vi "LBCB Operation Manager.vi"() -> ()   [LabVIEW 2009]
uses:
  lib/Data Display/External Sensor Name & Value.ctl
  lib/Data Access Objects/Application/App Parameters.ctl
  lib/Data Access Objects/Application/Timing Parameters.ctl
  lib/Apps/AppStates.ctl
  lib/Data Access Objects/Metadata/LBCB Number.ctl
  lib/Data Access Objects/Metadata/LBCB Location.ctl
  lib/Data Access Objects/Control Loop/PID Controls.ctl
  lib/Apps/Lbcb Control Loop States.ctl
  lib/MixedMode/Stiffness Matrix.ctl
  lib/MixedMode/Target Data.ctl
  lib/MixedMode/Mixed Mode Cartesian Data.ctl
  lib/MixedMode/Mixed Mode Convergence Status.ctl
  lib/Autobalance/Autobalance Display Data Point.ctl
  lib/Autobalance/Autobalance Stage.ctl
  lib/Apps/Yes No Button.ctl
  lib/Data Access Objects/Autobalance/Autobalance Control Parameters.ctl
  lib/Data Access Objects/Metadata/Actuator Point.ctl
  lib/Data Access Objects/Metadata/Cartesian Force Vector.ctl
  lib/Data Access Objects/Metadata/Cartesian Force Matrix.ctl
  lib/Data Access Objects/Mixed Mode/Force Control Parameters.ctl
  lib/Data Access Objects/Metadata/Cartesian Point.ctl
  lib/MixedMode/Mixed Mode States.ctl
  lib/MixedMode/Mixed Mode Multidof State.ctl
  lib/Apps/App Parameters Actions.ctl
  lib/Apps/App Status Actions.ctl
  lib/Apps/GUI Control.ctl
  lib/MixedMode/Messages/MM Widget Parameter Changes.ctl
  lib/Control Loop/Parameters Changes.ctl
  lib/Control Loop/Parameter Change States.ctl
  lib/MixedMode/Messages/Mixed Mode Command.ctl
  lib/MixedMode/Mixed Mode Command Action.ctl
  lib/MixedMode/Ramp Time Tuple.ctl
  lib/Data Access Objects/Metadata/Persistant DAO Actions.ctl
  lib/MixedMode/Messages/Mixed Mode Status.ctl
  lib/Data Access Objects/Metadata/DAO Actions.ctl
  lib/Data Access Objects/Application/Number Of LBCBs.ctl
  lib/Limits/Faults List Actions.ctl
  lib/Configuration/ConfigPathActions.ctl
  lib/Launcher/Launcher Actions.ctl
  lib/Logging/Log Filename Actions.ctl
  lib/Launcher/NoPanelAppTypes.ctl
  lib/Global Data/Actuator Measurment Actions.ctl
  lib/Logging/LogFileType.ctl
  lib/Global Data/Cartesian Measurment Actions.ctl
  lib/DAQ IO/Daq Actions.ctl
  lib/Control Loop/LBCB_Conversions_Actions.ctl
panel:
  out "Rigid Connection":T1
  in  "Snapshot":bool
  out "LBCB  Location Out":T2
  in  "Start AB Selected":bool
  in  "Start Autobalance":bool
  in  "Fake":bool
  out "LBCB 2 State":T3
  out "LBCB 1 State":T3
  in  "LBCB Number Button":bool
  in  "L2 Control":bool caption="LBCB 2"
  in  "L1 Control":bool caption="LBCB 1"
  out "L2 Force Limit":bool=TRUE caption="Force"
  out "L2 Displacement Limit":bool=TRUE caption="Displacement"
  out "L2 Auto Balance":bool=TRUE caption="Auto Balance"
  in  "PID Control":T4={"I-Control"=TRUE, "Ctrl Mode"=TRUE}
  in  "LBCB Number":T5
  out "State":T6=enum."Initializing Displays"
  out "Application Timing and Logging":T7
  out "External Sensor Names":string[](array[string])
  out "all stopped":bool
  out "Messages":string
  out "L1 Force Limit":bool=TRUE caption="Force"
  out "L1 Displacement Limit":bool=TRUE caption="Displacement"
  out "L1 Auto Balance":bool=TRUE caption="Auto Balance"
  in  "stop":bool
  in  "Monitor Panel":T9(tab)
  out "Cartesian DOF Labels":string[](array[string])=["X", "Y", "Z", "Rx", "Ry", "Rz"]
  out "Cartesian Space Labels":string[](array[string])=["Commands (in/rad)", "Displacements (in/rad)", "Forces (lbs/lb*in)"]
  out "External Sensors":T10[](array[typedef])
  out "Cartesian Digital Display Table":dbl[][](array[numeric])
  out "Actuator Digital Display":dbl[][](array[numeric])
  out "Actuator DOF Labels":string[](array[string])=["X1", "X2", "Y1", "Z1", "Z2", "Z3"]
  out "Actuator Space Labels":string[](array[string])=["Commands (in/rad)", "Displacements (in/rad)", "Forces (lbs/lb*in)"]
  out "Actuator X1":dbl(slide)=0.012801822908652838 step=0.0005 scale=-10.0..10.0
  out "Actuator X2":dbl(slide)=0.012801822908652838 step=0.0005 scale=-10.0..10.0
  out "Actuator Y1":dbl(slide)=7.98290599846041e-06 step=0.0005 scale=-5.0..5.0
  out "Actuator Z1":dbl(slide)=8.154359441903125e-06 step=0.0005 scale=-5.0..5.0
  out "Actuator Z2":dbl(slide)=8.154359441903125e-06 step=0.0005 scale=-5.0..5.0
  out "Actuator Z3":dbl(slide)=8.154359441903125e-06 step=0.0005 scale=-5.0..5.0
  in  "Cartesian Type":bool caption="Coord"
  out "External Sensors Volts":T10[](array[typedef]) caption="External Sensor Voltages"
  out "Actuator Labels":string[](array[string])=["X1", "X2", "Y1", "Z1", "Z2", "Z3"]
  out "Voltage Labels":string[](array[string])=["Commands", "LVDTs", "Load Cells", "Servo Errors"]
  out "Raw Data":dbl[][](array[numeric])
  in  "Force Error Range":T11
  in  "Jacobian Gain":T12
  in  "Max Increment":T12
  in  "Force Control Parameters":T13
  in  "Stiffness Limit":T14
  in  "Force Group Priorities":T11
  out "Convergence":T15
  out "Measurements":T16
  out "Target":T17
  in  "Stiffness Jacobian":T18=[[1000000.0, 0.0, 0.0, 0.0, 0.0, 0.0], [0.0, 1000000.0, 0.0, 0.0, 0.0, 0.0], [0.0, 0.0, 1000000.0, 0.0, 0.0, 0.0], [0.0, 0.0, 0.0, 1000000.0, 0.0, 0.0], [0.0, 0.0, 0.0, 0.0, 1000000.0, 0.0], [0.0, 0.0, 0.0, 0.0, 0.0, 1000000.0]]
  out "MixedModeStates":T19
  out "Mixed Mode Multidof State":T20
  out "MM Multi Ramp Count":i32 caption="Ramp Count"
  out "Stiffness Tested":T1[](array[typedef])
  in  "Auto Balance Error Window":T21
  in  "Auto Balance Control":T22={"Number of Samples"=0, "Delay After Cmd"=0, "Maximum Command"=0.0, "1/4 Linear Range"=0.5}
  out "Autobalance Statuses":T23[](array[typedef])
  out "Logo":picture
  # "Operations Manager"
  # "Ver 3.2.0"
  # "NEES MUST-SIM Facility"
  # "University of Illinois at Urbana-Champaign"
  # "Control"
  # "Continuous"
  # "Hold"
  # "Interval is in Seconds\nRate is in Samples per Second"
  # "(inch)"
  # "(inch)"
  # "(inch)"
  # "(inch)"
  # "(inch)"
  # "(inch)"
  # "Actuator\nSpace"
  # "Name"
  # "Cartesian\nSpace"
  # "Multi DOF\nStatus"
  # "(Volts)"
  # "Cmd"
  # "Servo Error"
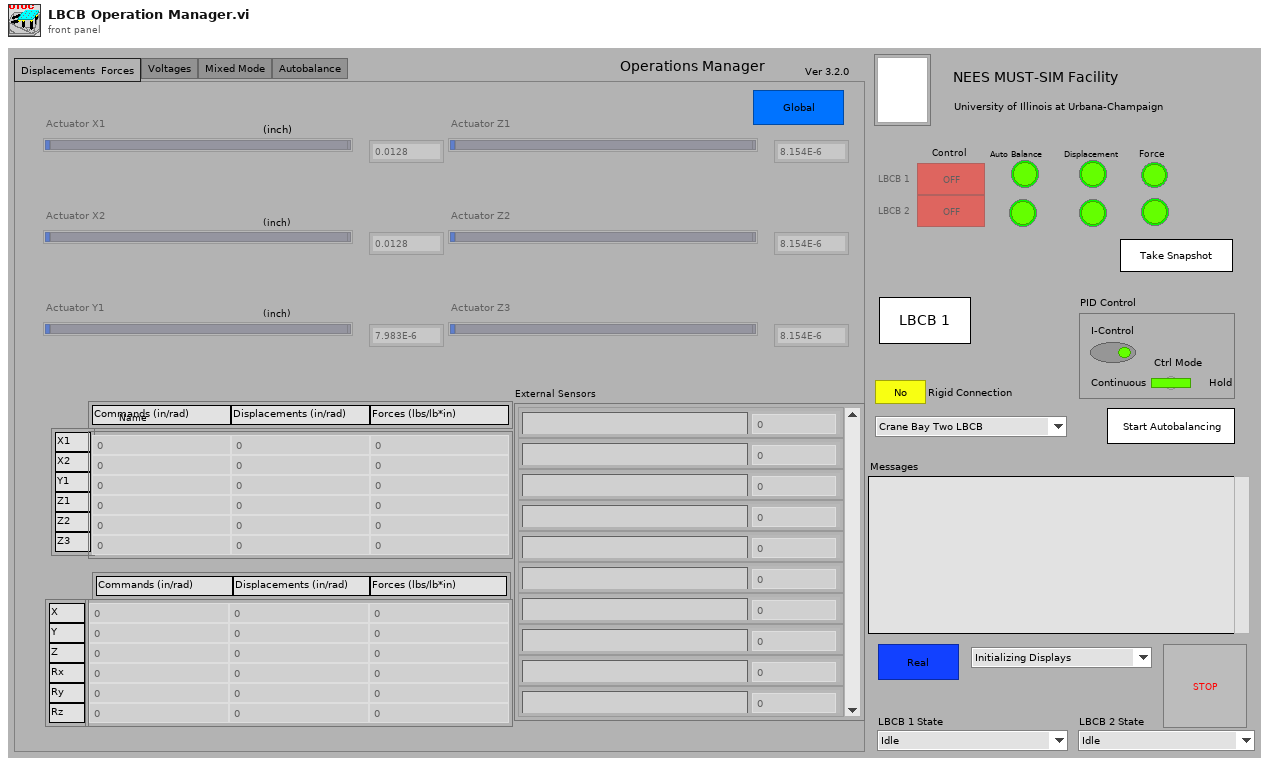
[diagram p1: front panel]
types:
  T1 = typedef "Yes No Button.ctl" = bool
  T2 = typedef "LBCB Location.ctl" = enum16{"Crane Bay Two LBCB", "Crane Bay One LBCB", "5th Scale Two LBCB", "5th Scale One LBCB", "Portable LBCB"}
  T3 = typedef "Lbcb Control Loop States.ctl" = enum16{"Idle", "Start Selected", "Load Last Command", "Start Autobalancing", "Autobalancing", "Control Loop Initialized", "Control Enabled"}
  T4 = typedef "PID Controls.ctl" = cluster{"I-Control":bool, "Ctrl Mode":bool}
  T5 = typedef "LBCB Number.ctl" = enum16{"LBCB1", "LBCB2"}
  T6 = typedef "AppStates.ctl" = enum16{"Starting OM", "Initializing Displays", "Setting up Archiving", "Setting Up DAQ Channels", "Start DAQ", "DAQ Starting", "Controlling LBCBs", "Stopping OM"}
  T7 = typedef "App Parameters.ctl" = cluster{"Monitor Loop":T8, "Ramp Time":T8, "Log Loop":T8, "TCP to DAQ":T8, "Logging Directory":path, "Log File Size (MBytes)":i64, "Volt Logging Loop":T8, "2 LBCB Archiving Mode":bool}
  T8 = typedef "Timing Parameters.ctl" = cluster{"Interval":dbl, "Rate ":dbl}
  T9 = enum32{"Displacements  Forces", "Voltages", "Mixed Mode", "Autobalance"}
  T10 = typedef "External Sensor Name & Value.ctl" = cluster{"Name":string, "Value":dbl}
  T11 = typedef "Cartesian Force Vector.ctl" = cluster{"Fx":dbl, "Fy":dbl, "Fz":dbl, "Mx":dbl, "My":dbl, "Mz":dbl}
  T12 = typedef "Cartesian Point.ctl" = cluster{"Dx":dbl, "Dy":dbl, "Dz":dbl, "Rx":dbl, "Ry":dbl, "Rz":dbl}
  T13 = typedef "Force Control Parameters.ctl" = cluster{"Use Force Error Range Ratios":bool, "Use Group Priorities":bool, "Multi Command Update":bool, "Steps per Stiffness \nMeasurement":i32}
  T14 = typedef "Cartesian Force Matrix.ctl" = cluster{"Lower":T11, "Upper":T11}
  T15 = typedef "Mixed Mode Convergence Status.ctl" = cluster{"IsConverged":bool[], "Force Errors":dbl[], "Controlling DOF":bool[]}
  T16 = typedef "Mixed Mode Cartesian Data.ctl" = cluster{"Displacements":dbl[], "Forces":dbl[]}
  T17 = typedef "Target Data.ctl" = cluster{"Displacements":dbl[], "Command Type":enum16{"<None>", "Displacement", "Force"}[], "Forces":dbl[]}
  T18 = typedef "Stiffness Matrix.ctl" = dbl[][]
  T19 = typedef "Mixed Mode States.ctl" = enum16{"Init", "Wait For DAQ", "Idle", "Start Initial Position", "Initial Position", "Start Initial Ramp", "Run Initial Ramp", "Start Iterative Stage", "Convergence Check", "Update Stiffness Jacobian", "Update Command", "Start Iterative Ramp", "Run Iterative Ramp", "Start Iterative Stabilize", "Iterative Stabilize", "Start Iterative Holding", "Iterative Holding", "Start Stabilize", "Stabilize", "Start Hold", "Holding", "Done", "Aborting", "Exit", "Nop"}
  T20 = typedef "Mixed Mode Multidof State.ctl" = enum16{"Multidof", "Stiffness Test", "Start Iterative Stage"}
  T21 = typedef "Actuator Point.ctl" = cluster{"X1":dbl, "X2":dbl, "Y1":dbl, "Z1":dbl, "Z2":dbl, "Z3":dbl}
  T22 = typedef "Autobalance Control Parameters.ctl" = cluster{"Number of Samples":i32, "Delay After Cmd":i32, "Maximum Command":dbl, "1/4 Linear Range":dbl}
  T23 = typedef "Autobalance Display Data Point.ctl" = cluster{"LoCmd":dbl, "LoServo":dbl, "HiCmd":dbl, "HiServo":dbl, "Autobalance Stage":T24, "IsBalanced":T1}
  T24 = typedef "Autobalance Stage.ctl" = enum16{"Coarse", "Fine", "Backing Up", "Done"}
  T25 = typedef "Mixed Mode Status.ctl" = cluster{"LBCB Target":T17[], "MixedModeStates":T19, "LBCB Convergence":T15[], "LBCB Measurements":T16[]}
  T26 = typedef "GUI Control.ctl" = cluster{"Command":T27, "LBCB Number":enum16{"LBCB1", "LBCB2"}}
  T27 = typedef "MM Widget Parameter Changes.ctl" = enum16{"Start", "Stop All", "Cartesian Type Changed", "Control Enabled", "Control Disabled", "NTCP Link On", "NTCP Link Off"}
  T28 = typedef "Persistant DAO Actions.ctl" = enum16{"Init", "Get", "Set", "Load", "Save"}
  T29 = typedef "Mixed Mode Command.ctl" = cluster{"Command":T30, "Ramp Times":cluster{"Initial":T31, "Iterative":T31}, "LBCB1":T17, "LBCB2":T17}
  T30 = typedef "Mixed Mode Command Action.ctl" = enum16{"Start Command", "Stop", "Exit", "No Op", "Start Acquisition", "Measure Initial Position"}
  T31 = typedef "Ramp Time Tuple.ctl" = cluster{"Ramp":dbl, "Stab":dbl, "Hold":dbl}
  T32 = typedef "Parameters Changes.ctl" = cluster{"Change State":T33, "LBCB Number":T5}
  T33 = typedef "Parameter Change States.ctl" = enum16{"Mixed Mode", "Control Loop", "Limits", "Application", "Stiffness Jacobian", "Start DAQ", "Reset Auto-Balance", "Set Command", "Enable Control", "Disable Control", "Position", "Stop Application"}
  T34 = typedef "App Status Actions.ctl" = enum16{"Init", "Get Status", "Running", "Control", "Autobalanced", "Data Acquisition", "Set App State", "DAQ Started", "Set LBCB State", "Set All", "Set Cont Logging", "Set Step Logging", "Set MM Logging", "Set Volt Logging", "Set Cart Type", "Set DAQ Link", "Set NTCP Link"}
  T35 = enum8{"Enabled", "Disabled", "Disabled and Grayed Out"}
  T36 = typedef "Number Of LBCBs.ctl" = enum16{"1", "2"}
  T37 = typedef "LBCB Settings.ctl" = cluster{"Size":T38, "Type":T39}
  T38 = typedef "LBCB Size.ctl" = enum16{"1/5th-scale LBCB", "Full-scale LBCB", "Portable LBCB"}
  T39 = typedef "LBCB Type.ctl" = enum16{"X Actuators On The Left", "X Actuators On The Right"}
  T40 = typedef "App Parameters Actions.ctl" = enum16{"Init", "Get", "Set"}
  T41 = typedef "DAO Actions.ctl" = enum16{"Init", "Get", "Set"}
  T42 = typedef "NoPanelAppTypes.ctl" = enum16{"NTCP Socket", "Data Archiving", "DAQ Link", "Control Loops", "Cmd Disp Diffs", "Individual Readings", "Limits", "Increment Limits"}
  T43 = typedef "Launcher Actions.ctl" = enum16{"Launch", "Stop All", "Stop", "Kill", "Running?", "Init"}
  T44 = typedef "Cartesian Matrix.ctl" = cluster{"Lower":T12, "Upper":T12}
  T45 = typedef "Faults List Actions.ctl" = enum16{"Init", "Add", "Remove", "Get List"}
  T46 = typedef "ConfigPathActions.ctl" = enum16{"Init", "Application", "MixedMode", "ControlLoop", "Calibration", "System", "Change Location"}
  T47 = typedef "Log Filename Actions.ctl" = enum16{"Init", "Get Filename", "New Log Directory"}
  T48 = typedef "Actuator Measurment Actions.ctl" = enum16{"Set  Data", "Get", "Init"}
  T49 = typedef "LogFileType.ctl" = enum16{"Continuous", "Step", "Volts", "Offsets", "Mixed Mode State", "DLL  Errors", "Snapshot", "End List"}
  T50 = typedef "Daq Actions.ctl" = enum16{"Init", "Send Commands", "Get Responses", "Stop"}
  T51 = typedef "LBCB_Conversions_Actions.ctl" = enum16{"A2C", "C2A", "Set Log Filename", "Init"}
  T52 = typedef "App Status.ctl" = cluster{"Running":bool, "Controlling L2":bool, "Autobalance L2":bool, "Data Acquisition":bool, " App State":T6, "DAQ Started":bool, "LBCB 1 State":T3, "LBCB 2 State":T3, "Controlling L1":bool, "Autobalance L1":bool, "Cartesian Type":bool, "Continuous Logging":bool, "Step Logging":bool, "Voltage Logging":bool, "Mixed Mode Logging":bool, "DAQ Link":bool, "NTCP Link ":bool}
  T53 = typedef "Limit Boundary Parameters.ctl" = cluster{"Lower":dbl, "Upper":dbl, "Label":string}
  T54 = typedef "imagedata.ctl" = cluster{"image type":i32, "image depth":i32, "image":u8[], "mask":u8[], "colors":u32[], "Rectangle":cluster{"left":i16, "top":i16, "right":i16, "bottom":i16}}
  T55 = typedef "Cartesian Measurment Actions.ctl" = enum16{"Set Data", "Get", "Init", "Set Offsets"}
  T56 = typedef "Actuator DataType.ctl" = cluster{"LVDTs":dbl[], " Commands":dbl[], "Load Cells":dbl[], "Servo":dbl[]}
  T57 = typedef "Mixed Mode Multidof Status.ctl" = cluster{"Mixed Mode Multidof State":T20, "Multi DOF Ramp Count":i32, "Stiffness Tested":T1[][]}
  T58 = typedef "Autobalance Status Data.ctl" = cluster{"IsBalanced":T1, "Autobalance Stage":T24, "High":T59, "Low":T59, "Balanced \nCmd":dbl}
  T59 = typedef "Autobalance Data Point.ctl" = cluster{"cCmd":dbl, "cServo":dbl, "pCmd":dbl, "pServo":dbl}
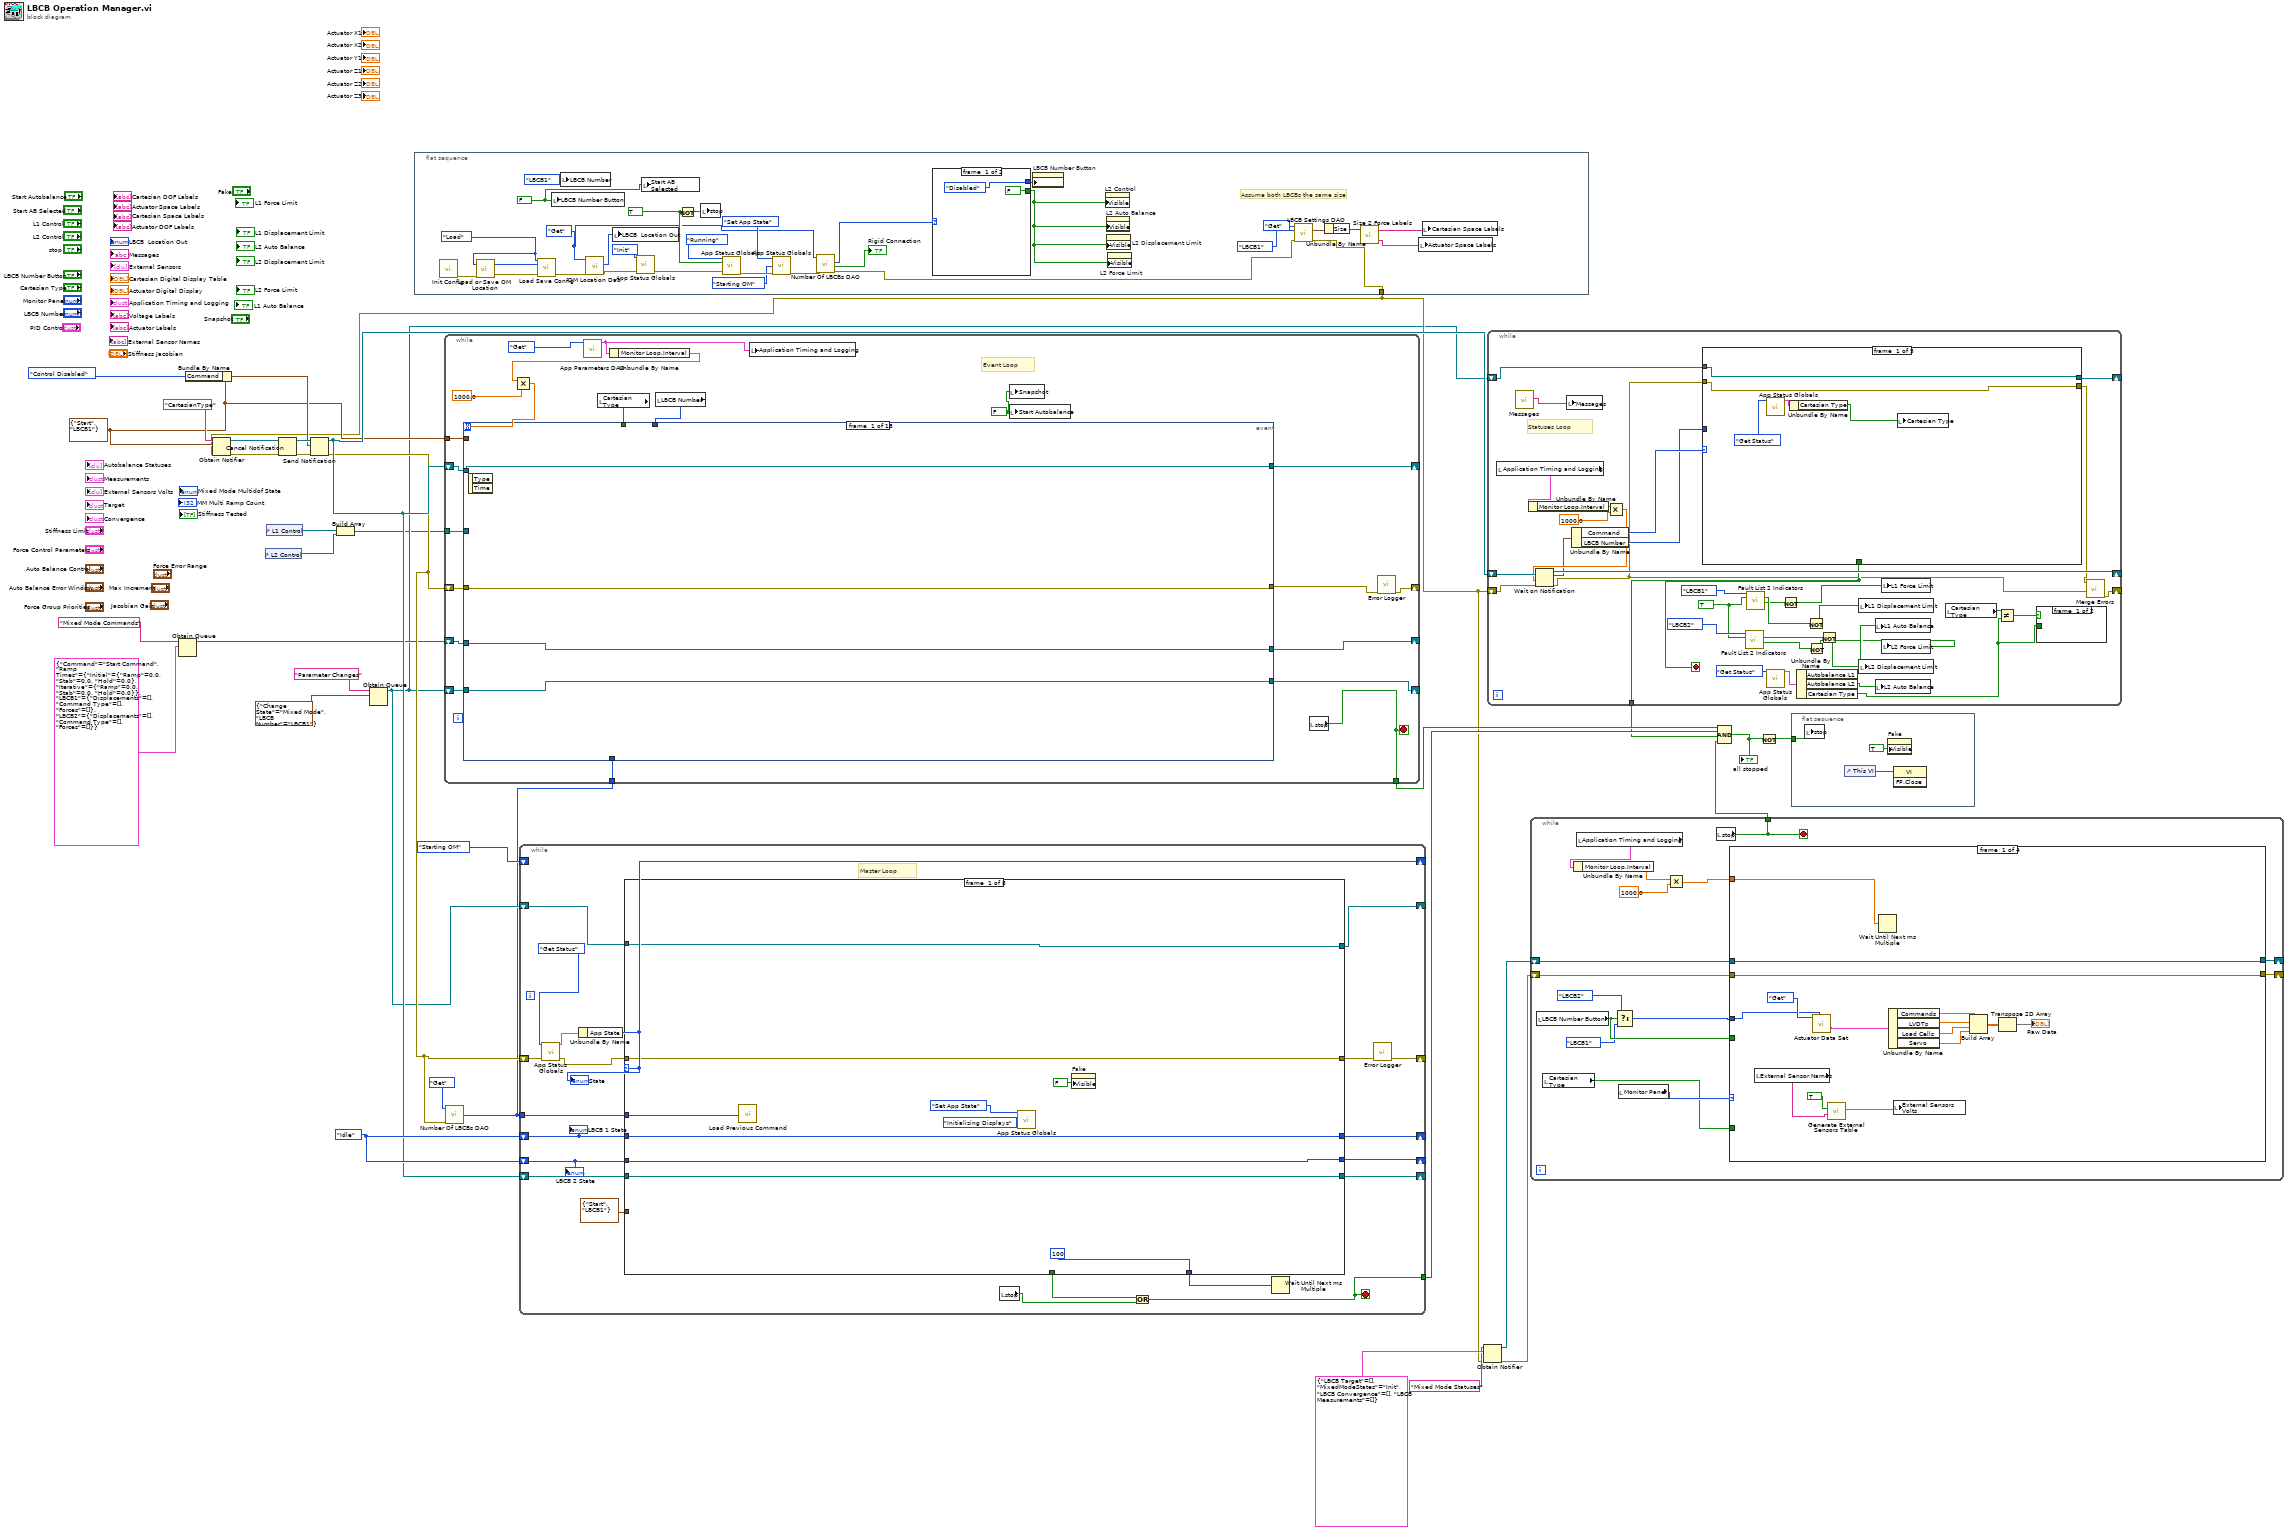
[diagram p0: block diagram]
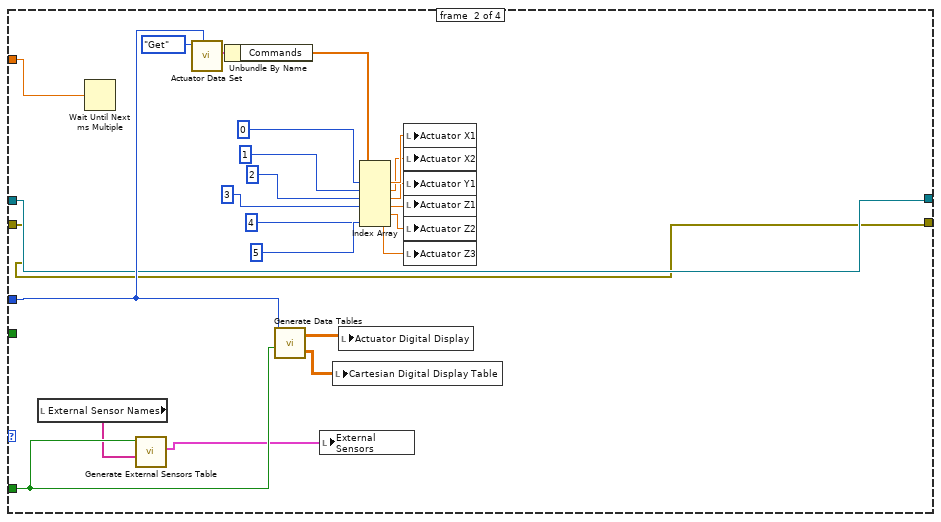
[diagram p2: hidden frame]
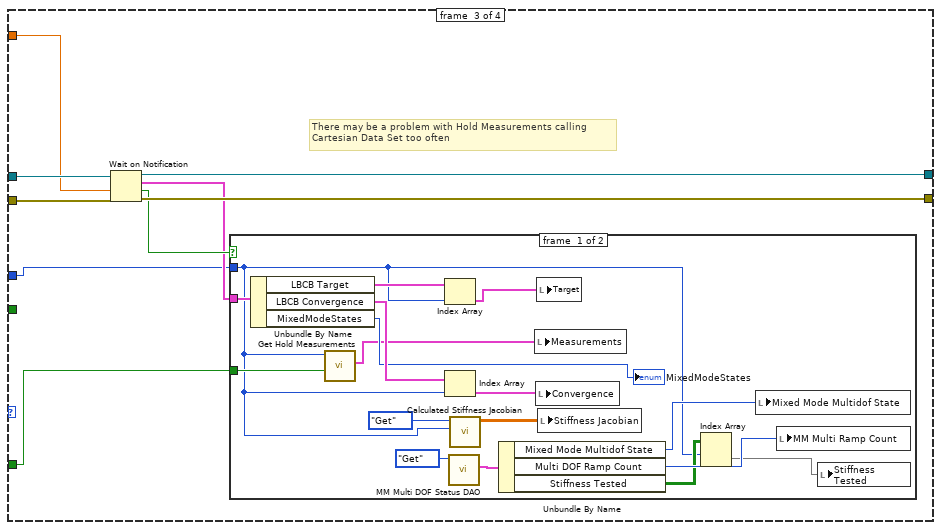
[diagram p3: hidden frame]
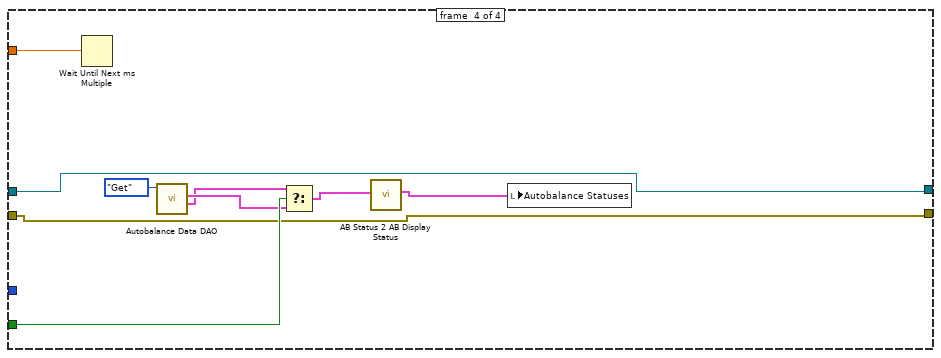
[diagram p5: hidden frame]
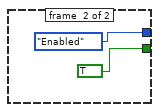
[diagram p6: hidden frame]
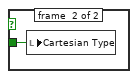
[diagram p7: hidden frame]
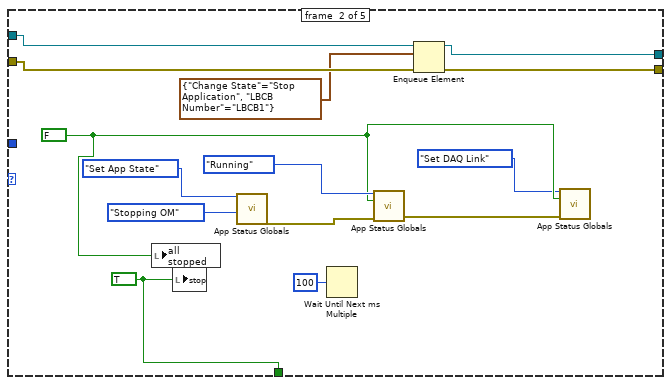
[diagram p8: hidden frame]
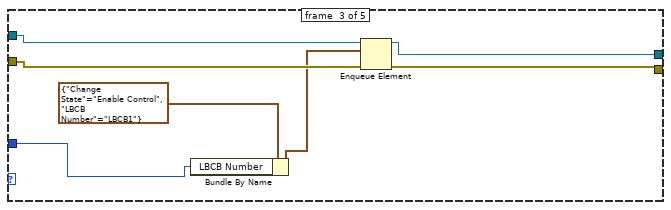
[diagram p9: hidden frame]
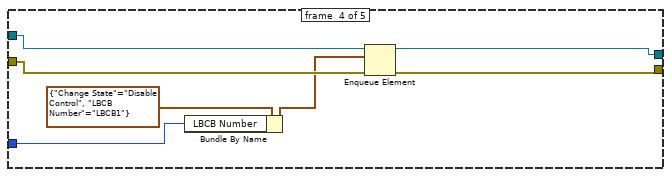
[diagram p10: hidden frame]
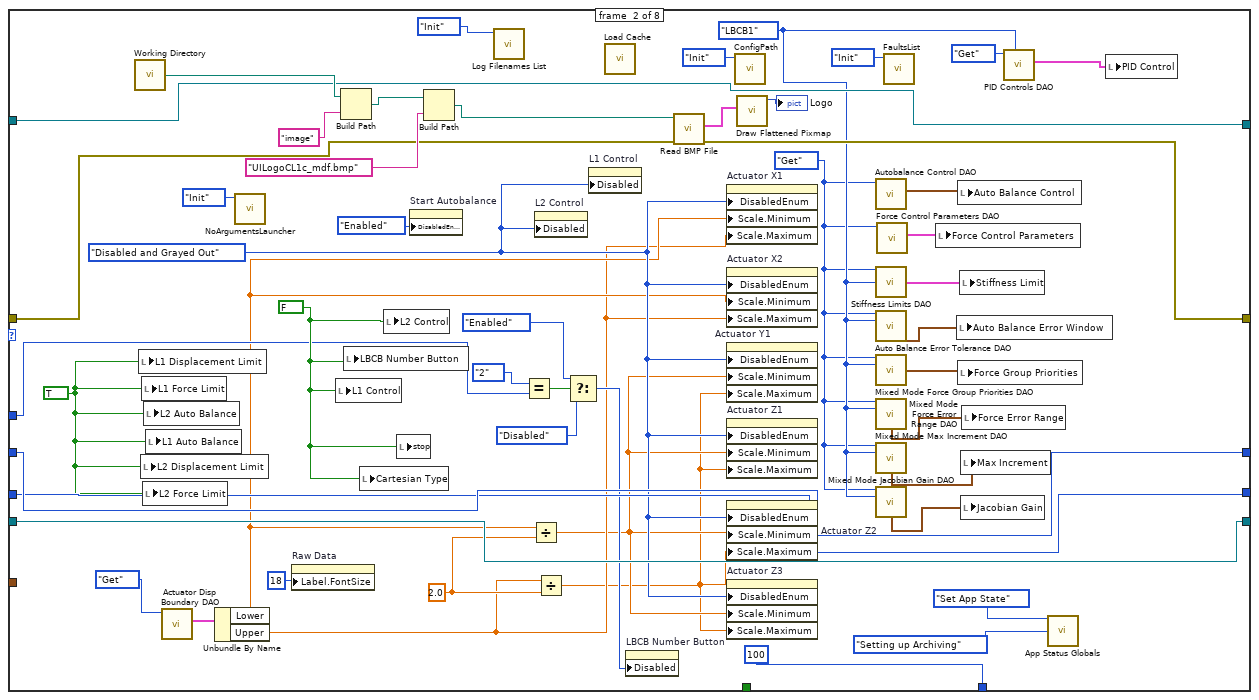
[diagram p12: hidden frame]
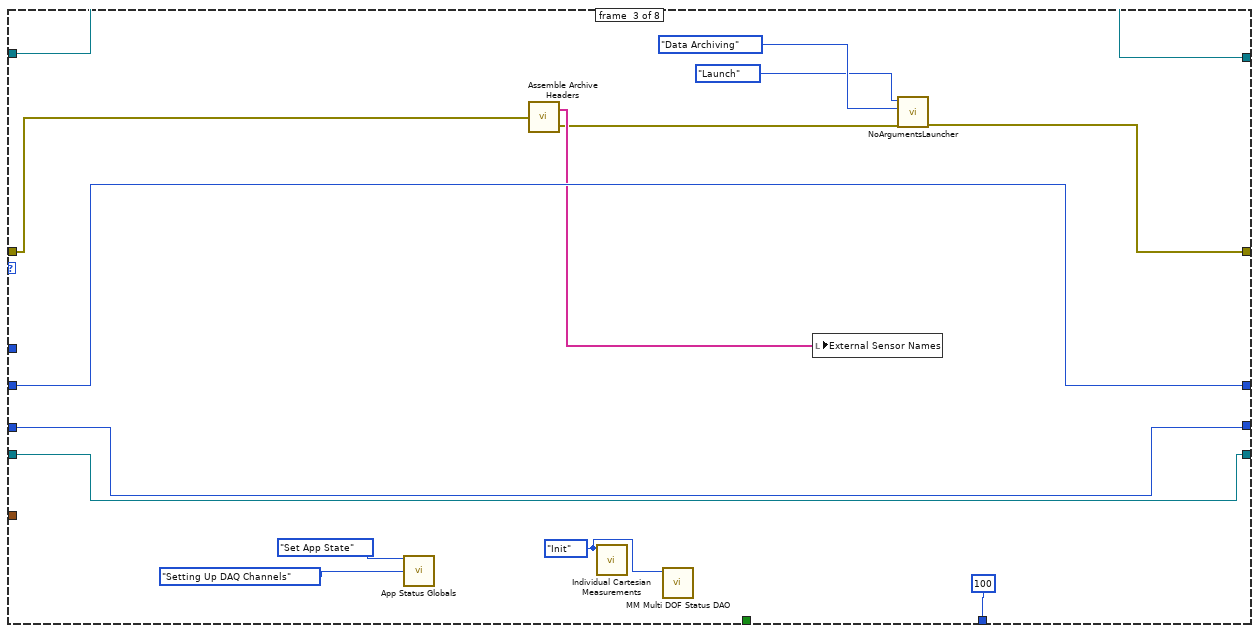
[diagram p13: hidden frame]
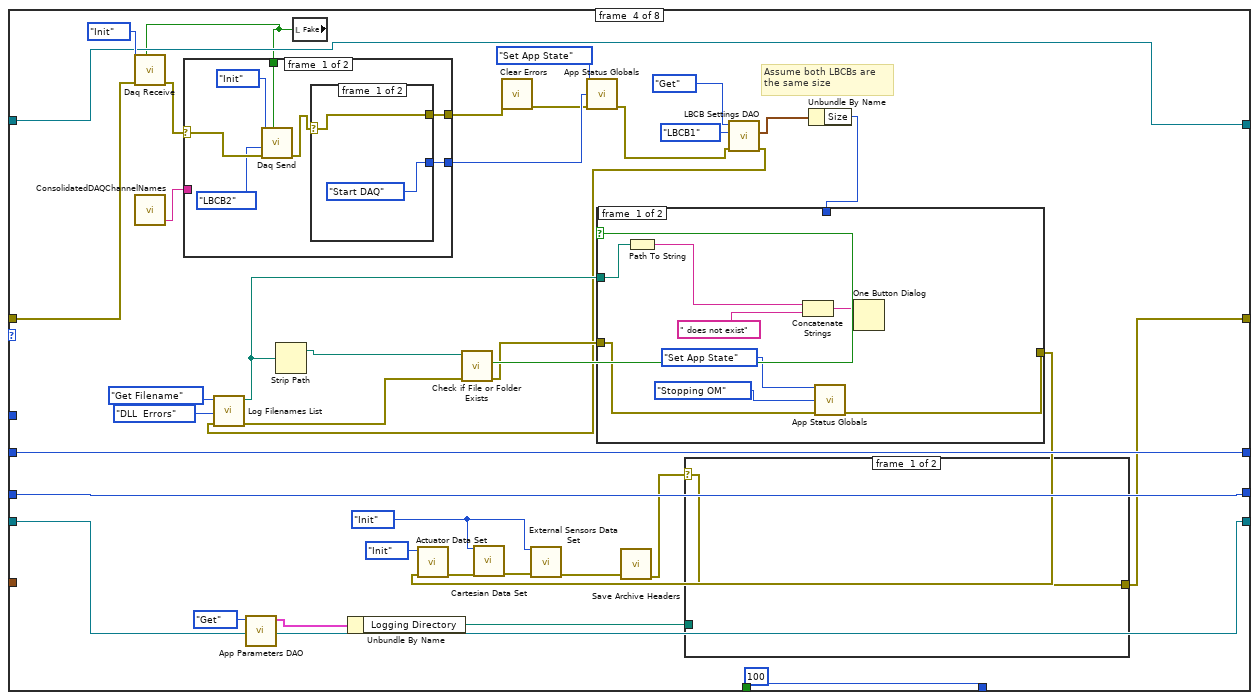
[diagram p14: hidden frame]
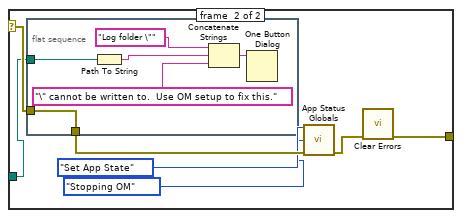
[diagram p15: hidden frame]
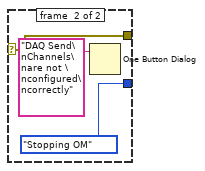
[diagram p16: hidden frame]
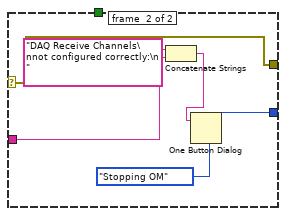
[diagram p17: hidden frame]
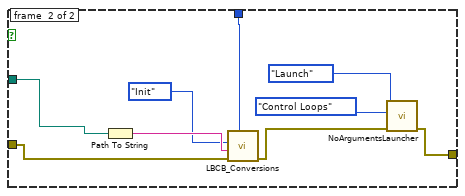
[diagram p18: hidden frame]
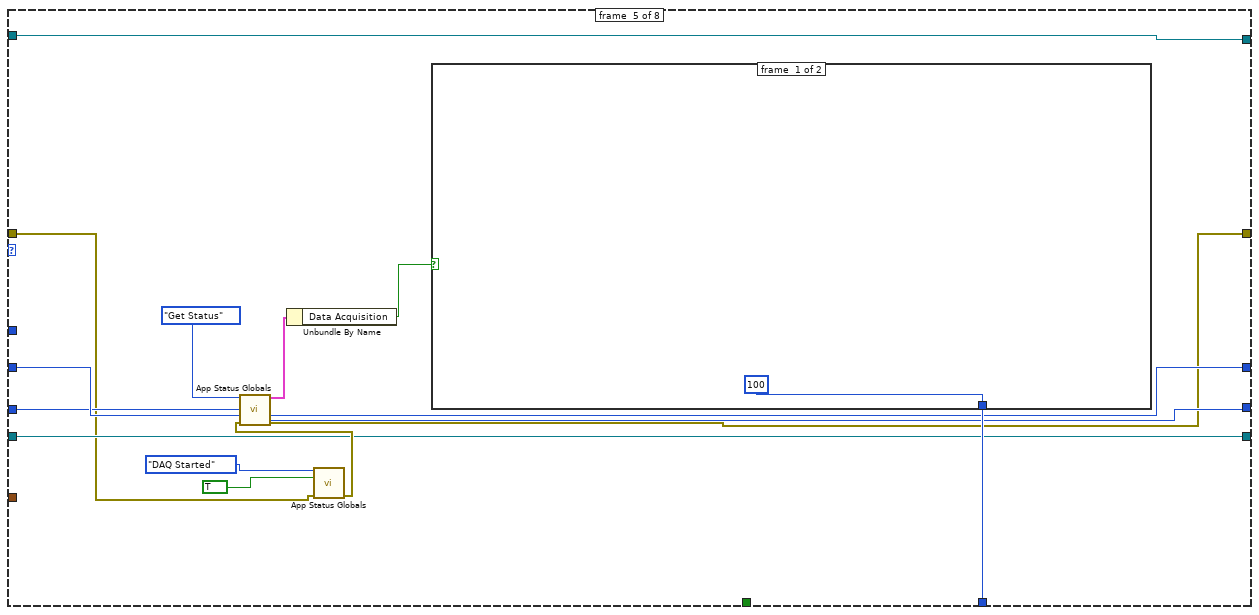
[diagram p19: hidden frame]
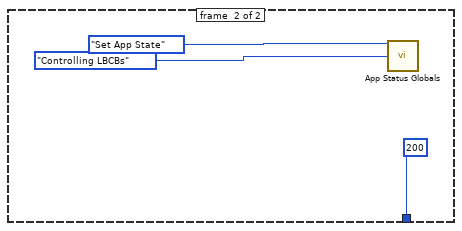
[diagram p20: hidden frame]
diagram:
  w13 = T26 {"Command"=enum."Start", "LBCB Number"=enum."LBCB1"} ("GUI Control")
  w26 = Lbcb_Control_Loop_States."Idle" ("f")
  n1 = Obtain Queue(name (unnamed)="Mixed Mode Commands", element data type=T29 {"Command"=enum."Start Command", "Ramp Times"={"Initial"={"Ramp"=0.0, "Stab"=0.0, "Hold"=0.0}, "Iterative"={"Ramp"=0.0, "Stab"=0.0, "Hold"=0.0}}, "LBCB1"={"Displacements"=[], "Command Type"=[], "Forces"=[]}, "LBCB2"={"Displacements"=[], "Command Type"=[], "Forces"=[]}} ("Mixed Mode Command")) -> (queue out=w6:refnum<queue>)  [unwired: 3 in, 2 out]
  n2 = Bundle By Name(cluster=w13, "Command"=MM_Widget_Parameter_Changes."Control Disabled" ("notification")) -> (w15:T26)
  n3 = Obtain Notifier(name (unnamed)="CartesianType", notification data type=w13, error in (no error)=w7) -> (notifier out=w34:refnum<notifier>, error out=w18:errorcluster)  [unwired: 1 in, 1 out]
  n4 = control-ref of="L2 Control"() -> (w3:refnum<vi>)
  n5 = control-ref of="L1 Control"() -> (w4:refnum<vi>)
  n6 = Cancel Notification(0:w34, 3:w18) -> (8:w20:refnum<notifier>, 11:w17:errorcluster)  [unwired: 1 out]
  n7 = Send Notification(notification=w15, notifier=w20, error in (no error)=w17) -> (notifier out=w19:refnum<notifier>, error out=w16:errorcluster)
  n8 = Build Array(w4, w3) -> (w2:refnum<vi>[])
  n9 = Obtain Queue(name (unnamed)="Parameter Changes", element data type=T32 {"Change State"=enum."Mixed Mode", "LBCB Number"=enum."LBCB1"} ("Parameter Changes")) -> (queue out=w5:refnum<queue>)  [unwired: 3 in, 2 out]
  n10 = flat-sequence {
    tunnel: [w37] -> w7
    frame #0 {
      w49 = FALSE ("LBCB Number Button")
      w47 = Persistant_DAO_Actions."Get" ("Actions")
      w59 = Persistant_DAO_Actions."Load" ("Actions")
      w51 = TRUE ("Status\nSetting")
      # "Assume both LBCBs the same size"
      n11 = call "Init Config.vi"() -> ("error out"=w54:errorcluster)  [unwired: 1 in, 10 out]
      n12 = call "Load or Save OM Location.vi"("error in (no error)"=w54, "Action"=w59) -> ("error out"=w60:errorcluster, "LBCB  Location Out"=w52:T2)
      n13 = call "Load Save Config.vi"("error in (no error)"=w60, "OM  Location"=w52, "Actions"=w59) -> ("error out"=w57:errorcluster)  [unwired: 8 out]
      n14 = local write "LBCB Number Button"(w49) -> ()
      n15 = local write "LBCB Number"(LBCB_Number."LBCB1" ("LBCB Number")) -> ()
      n16 = call "OM Location Dao.vi"("error in (no error)"=w57, "Actions"=w47) -> ("error out"=w58:errorcluster, "LBCB  Location Out"=w56:T2)  [unwired: 2 in, 6 out]
      n17 = local write "LBCB  Location Out"(w56) -> ()
      n18 = call "App Status Globals.vi"("App Status Actions"=App_Status_Actions."Init", "error in (no error)"=w58) -> ("error out"=w62:errorcluster)  [unwired: 5 in, 8 out]
      n19 = local write "Start AB Selected"(w49) -> ()
      n20 = Not(x=w51) -> (.not. x?=w53:bool)
      n21 = local write "stop"(w53) -> ()
      n22 = call "App Status Globals.vi"("App Status Actions"=App_Status_Actions."Running", "Status\nSetting"=w51, "error in (no error)"=w62) -> ("error out"=w64:errorcluster)  [unwired: 4 in, 8 out]
      n23 = call "App Status Globals.vi"("App Status Actions"=App_Status_Actions."Set App State", "App State"=AppStates."Starting OM" ("State"), "error in (no error)"=w64) -> ("error out"=w48:errorcluster)  [unwired: 4 in, 8 out]
      n24 = call "Number Of LBCBs DAO.vi"("error in (no error)"=w48, "Actions"=w47) -> ("error out"=w38:errorcluster, "Rigid Connection Out"=→"Rigid Connection":bool, "Number of\nLBCBs Out"=w46:T36)  [unwired: 6 in, 1 out]
      n25 = case shown="\"1\", Default" w46 {
        tunnel: [T35."Disabled" ("f") T35."Enabled" ("Disabled")] -> w45
        tunnel: [FALSE TRUE] -> w44
        frame #0 {
        }
        frame #1 {
        }
      }
      n26 = property on="LBCB Number Button" class="Bool (strict)"("DisabledEnum"=w45) -> ()  [unwired: 2 in, 2 out]
      n27 = property on="L2 Control" class="Bool (strict)"("Visible"=w44) -> ()  [unwired: 2 in, 2 out]
      n28 = property on="L2 Auto Balance" class="Bool (strict)"("Visible"=w44) -> ()  [unwired: 2 in, 2 out]
      n29 = property on="L2 Displacement Limit" class="Bool (strict)"("Visible"=w44) -> ()  [unwired: 2 in, 2 out]
      n30 = property on="L2 Force Limit" class="Bool (strict)"("Visible"=w44) -> ()  [unwired: 2 in, 2 out]
      n31 = call "LBCB Settings DAO.vi"("error in (no error)"=w38, "LBCB Number"=LBCB_Number."LBCB1", "Actions"=Persistant_DAO_Actions."Get") -> ("error out"=w37:errorcluster, "LBCB Setting Out"=w41:T37)  [unwired: 6 in, 1 out]
      n32 = Unbundle By Name(w41) -> ("Size"=w42:T38)
      n33 = call "Size 2 Force Labels.vi"("Size"=w42) -> ("Actuator Space Labels"=w35:string[], "Cartesian Space Labels In"=w36:string[])  [unwired: 1 in]
      n34 = local write "Actuator Space Labels"(w35) -> ()
      n35 = local write "Cartesian Space Labels"(w36) -> ()
    }
  }
  n36 = call "Number Of LBCBs DAO.vi"("error in (no error)"=w16, "Actions"=Persistant_DAO_Actions."Get") -> ("Number of\nLBCBs Out"=w1:T36)  [unwired: 3 in, 6 out]
  n37 = while {
    shift-right: [w85] -> _
    shift-left: w19 -> [w86]
    shift-right: [w81] -> _
    shift-left: w16 -> [w84]
    tunnel: [w76] -> w32
    shift-right: [w79] -> _
    shift-left: w5 -> [w80]
    shift-right: [w74] -> _
    shift-left: w6 -> [w75]
    tunnel: w13 -> [w73]
    tunnel: w2 -> [w72]
    tunnel: w1 -> [w71]
    stop <- w76 stop-if-true
    w70 = FALSE ("Start Autobalance")
    # "Event Loop"
    n38 = call "App Parameters DAO.vi"("Actions"=App_Parameters_Actions."Get" ("App Parameter Actions")) -> ("Application Timing and Logging Out"=w77:T7)  [unwired: 3 in, 7 out]
    n39 = local read "Cartesian Type"() -> (w83:bool)
    n40 = Unbundle By Name(w77) -> ("Monitor Loop.Interval"=w88:dbl)
    n41 = Multiply(x=w88, y=1000.0) -> (x*y=w87:dbl)
    n42 = local read "LBCB Number"() -> (w78:T5)
    n43 = event shown="[1] Menu Selection (User)" {
      selector: _ -> [_ _ _ _ _ _ _ _ _ _ _ _ _ _ _ _ _ _]
      dyn-events: _ -> [_ _ _ _ _ _ _ _ _ _ _ _ _ _ _ _ _ _]
      timeout: w87 -> [_ _ _ _ _ _ _ _ _ _ _ _ _ _ _ _ _ _]
      tunnel: w86 -> [w93 w102 w118 w146 w157 w166 w183 w198 w213 w228 w240 w252 w264 w276 w288 w300 w312 w319]
      tunnel: [w93 w102 w117 w145 w156 w166 w183 w198 w213 w228 w240 w252 w264 w276 w288 w300 w312 w319] -> w85
      tunnel: w84 -> [w94 w100 w115 w148 w158 w163 w185 w195 w208 w226 w238 w250 w262 w274 w286 w298 w310 w317]
      tunnel: [w94 w101 w116 w147 w158 w159 w182 w194 w215 w230 w242 w254 w266 w278 w290 w302 w306 w315] -> w82
      tunnel: w83 -> [_ _ w105 _ _ _ _ _ _ _ _ _ _ _ _ _ _ _]
      tunnel: w80 -> [w91 w99 w112 w142 w154 w164 w186 w196 w217 w232 w244 w256 w268 w280 w292 w304 w307 w314]
      tunnel: [w91 w98 w112 w142 w154 w164 w186 w196 w214 w229 w241 w253 w265 w277 w289 w301 w307 w314] -> w79
      tunnel: w78 -> [_ w97 w108 _ _ _ _ _ w209 w219 w235 w247 w259 w271 w283 w295 w309 _]
      tunnel: w75 -> [w92 w96 w113 w149 w155 w165 w187 w197 w216 w231 w243 w255 w267 w279 w291 w303 w313 w320]
      tunnel: [w92 w96 w113 w149 w155 w165 w187 w197 w216 w231 w243 w255 w267 w279 w291 w303 w313 w320] -> w74
      tunnel: w73 -> [_ _ w110 w144 w153 _ _ _ _ _ _ _ _ _ _ _ _ _]
      tunnel: w72 -> [_ _ _ w141 _ _ _ _ _ _ _ _ _ _ _ _ _ _]
      tunnel: w71 -> [_ _ _ _ _ _ _ _ _ _ _ _ _ _ _ _ _ _]
      event #0 {
        n44 = event-data() -> ()  [unwired: 3 out]
      }
      event #1 {
        n45 = event-data() -> ("ItemTag"=w103:string, "MenuRef"=w95:refnum<k9>)  [unwired: 1 out]
        n46 = call "Menu Actions.vi"("queue in"=w99, "LBCB Number"=w97, "menu reference"=w95, "error in"=w100, "ItemTag"=w103) -> ("queue out"=w98:refnum<queue>, "error out"=w101:errorcluster)
      }
      event #2 {
        # "Cartesian Type\nT = Local\nF = Global"
        n47 = event-data() -> ()  [unwired: 3 out]
        n48 = Not(x=w105) -> (.not. x?=w106:bool)
        n49 = call "App Status Globals.vi"("App Status Actions"=App_Status_Actions."Set Cart Type", "Status\nSetting"=w106, "error in (no error)"=w115) -> ("error out"=w114:errorcluster)  [unwired: 3 in, 9 out]
        n50 = Bundle By Name(cluster=w110, "LBCB Number"=w108, "Command"=MM_Widget_Parameter_Changes."Cartesian Type Changed" ("notification")) -> (w107:T26)
        n51 = Send Notification(notification=w107, notifier=w118, error in (no error)=w114) -> (notifier out=w117:refnum<notifier>, error out=w116:errorcluster)
        n52 = event-data("Discard?"=TRUE) -> ()  [unwired: 4 in, 1 out]
      }
      event #3 {
        n53 = event-data() -> ("CtlRef"=w140:refnum<vi>, "NewVal"=w121:bool)  [unwired: 1 out]
        n54 = Search 1D Array(1D array=w141, element=w140) -> (index of element=w137:i32)  [unwired: 1 in]
        n55 = Equal?(x=w137, y=0) -> (x = y?=w124:bool)
        n56 = Select(t=LBCB_Number."LBCB1" ("LBCB Number"), s=w124, f=LBCB_Number."LBCB2") -> (s? t:f=w133:T5)
        n57 = call "App Status Globals.vi"("App Status Actions"=App_Status_Actions."Control", "LBCB Number"=w133, "Status\nSetting"=w121) -> ()  [unwired: 4 in, 9 out]
        n58 = Select(t=MM_Widget_Parameter_Changes."Control Enabled" ("notification"), s=w121, f=MM_Widget_Parameter_Changes."Control Disabled") -> (s? t:f=w130:T27)
        n59 = Bundle By Name(cluster=w144, "Command"=w130, "LBCB Number"=w133) -> (w138:T26)
        n60 = Select(t=Lbcb_Control_Loop_States."Control Enabled" ("LBCB State"), s=w121, f=Lbcb_Control_Loop_States."Control Loop Initialized") -> (s? t:f=w128:T3)
        n61 = Send Notification(notification=w138, notifier=w146, error in (no error)=w148) -> (notifier out=w145:refnum<notifier>, error out=w147:errorcluster)
        n62 = call "App Status Globals.vi"("App Status Actions"=App_Status_Actions."Set LBCB State", "LBCB Number"=w133, "LBCB State"=w128) -> ()  [unwired: 4 in, 9 out]
        n63 = local read "L1 Control"() -> (w125:bool)
        n64 = local read "L2 Control"() -> (w126:bool)
        n65 = Select(t=w126, s=w124, f=w125) -> (s? t:f=w122:bool)
        n66 = Or(x=w122, y=w121) -> (x .or. y?=w120:bool)
        n67 = Select(t=T35."Disabled and Grayed Out" ("Disabled"), s=w120, f=T35."Enabled") -> (s? t:f=w123:T35)
        n68 = property on="Start Autobalance" class="Bool (strict)"("DisabledEnum"=w123) -> ()  [unwired: 2 in, 2 out]
      }
      event #4 {
        n69 = event-data() -> ()  [unwired: 4 out]
        n70 = Bundle By Name(cluster=w153, "Command"=MM_Widget_Parameter_Changes."Stop All" ("notification")) -> (w151:T26)
        n71 = Send Notification(notification=w151, notifier=w157) -> (notifier out=w156:refnum<notifier>)  [unwired: 1 in, 1 out]
      }
      event #5 {
        n72 = event-data() -> ()  [unwired: 4 out]
        n73 = call "Snapshot"("error in (no error)"=w163) -> ("Snapshot"=w161:string, "OK"=w160:bool, "error out"=w162:errorcluster)  [unwired: 16 in]
        n74 = case shown="True" w160 {
          tunnel: w162 -> [w167 w170]
          tunnel: w161 -> [_ w169]
          tunnel: [w167 w168] -> w159
          frame #0 {
          }
          frame #1 {
            n75 = call "Take Snapshot.vi"("error in (no error)"=w170, "Snapshot Label"=w169) -> ("error out"=w168:errorcluster)  [unwired: 9 in]
          }
        }
      }
      event #6 {
        w179 = Persistant_DAO_Actions."Get" ("DAO Actions")
        n76 = event-data() -> ("NewVal"=w184:bool)  [unwired: 1 out]
        n77 = flat-sequence {
          tunnel: w184 -> [w192]
          tunnel: w185 -> [w189]
          tunnel: [w189] -> w182
          tunnel: [w188] -> w178
          frame #0 {
            n78 = Select(t=LBCB_Number."LBCB2", s=w192, f=LBCB_Number."LBCB1" ("LBCB Number")) -> (s? t:f=w188:T5)
            n79 = local write "LBCB Number"(w188) -> ()
          }
        }
        n80 = call "PID Controls DAO.vi"("LBCB Number"=w178, "Actions"=DAO_Actions."Get") -> ("PID Control  Out"=w181:T4)  [unwired: 8 in, 1 out]
        n81 = call "Force Control Parameters DAO.vi"("DAO Actions"=w179) -> ("Force Control Parameters Out"=w177:T13)  [unwired: 8 in, 2 out]
        n82 = call "Stiffness Limits DAO.vi"("Cartesian Force Limit Actions"=w179, "ID"=w178) -> ("Stiffness Limit Out"=w176:T44)  [unwired: 11 in, 2 out]
        n83 = call "Auto Balance Error Tolerance DAO.vi"("Auto Balance Increment Actions"=w179, "LBCB Number"=w178) -> ("Auto Balance Error Out"=w175:T21)  [unwired: 11 in, 2 out]
        n84 = call "Mixed Mode Force Group Priorities DAO.vi"("Force Error Range Actions"=w179, "LBCB Number"=w178) -> ("Force Group Priorities Out"=w171:T11)  [unwired: 11 in, 2 out]
        n85 = call "Mixed Mode Force Error Range DAO.vi"("Force Error Range Actions"=w179, "LBCB Number"=w178) -> ("Force Error Range Out"=w174:T12)  [unwired: 11 in, 2 out]
        n86 = call "Mixed Mode Max Increment DAO.vi"("Max Increment Actions"=w179, "LBCB Number"=w178) -> ("Max Increment Out"=w173:T12)  [unwired: 11 in, 2 out]
        n87 = call "Mixed Mode Jacobian Gain DAO.vi"("Jacobian Gain Actions"=w179, "LBCB Number"=w178) -> ("Jacobian Gain Out"=w172:T12)  [unwired: 11 in, 2 out]
        n88 = local write "Auto Balance Error Window"(w175) -> ()
        n89 = local write "Force Control Parameters"(w177) -> ()
        n90 = local write "Stiffness Limit"(w176) -> ()
        n91 = local write "Force Group Priorities"(w171) -> ()
        n92 = local write "PID Control"(w181) -> ()
        n93 = local write "Max Increment"(w173) -> ()
        n94 = local write "Jacobian Gain"(w172) -> ()
        n95 = local write "Force Error Range"(w174) -> ()
      }
      event #7 {
        n96 = event-data() -> ()  [unwired: 3 out]
        n97 = local read "L2 Control"() -> (w199:bool)
        n98 = local read "L1 Control"() -> (w200:bool)
        n99 = Compound Arithmetic op=AND(invert w200, invert w199) -> (w193:bool)
        n100 = case shown="True" w193 {
          tunnel: w193 -> [_ w206]
          tunnel: w195 -> [w201 w203]
          tunnel: [w201 w202] -> w194
          frame #0 {
          }
          frame #1 {
            n101 = local write "Start AB Selected"(w206) -> ()
            n102 = call "NoArgumentsLauncher.vi"("error in (no error)"=w203, "Application"=NoPanelAppTypes."Cmd Disp Diffs", "Application Launcher Actions"=Launcher_Actions."Launch") -> ("error out"=w202:errorcluster)  [unwired: 8 out]
          }
        }
      }
      event #8 {
        n103 = event-data() -> ("NewVal"=w210:T4)  [unwired: 1 out]
        n104 = call "PID Controls DAO.vi"("LBCB Number"=w209, "error in (no error)"=w208, "PID Control In"=w210, "Actions"=DAO_Actions."Set") -> ("error out"=w207:errorcluster)  [unwired: 6 in, 1 out]
        n105 = Bundle By Name(cluster=T32 {"Change State"=enum."Control Loop", "LBCB Number"=enum."LBCB1"} ("element"), "LBCB Number"=w209) -> (w212:T32)
        n106 = Enqueue Element(queue=w217, element=w212, error in (no error)=w207) -> (queue out=w214:refnum<queue>, error out=w215:errorcluster)  [unwired: 2 out]
      }
      event #9 {
        n107 = event-data() -> ("NewVal"=w224:T18)  [unwired: 1 out]
        n108 = call "Calculated Stiffness Jacobian.vi"("error in (no error)"=w226, "Stiffness Jacobian In"=w224, "LBCB Number"=w219, "Actions"=Persistant_DAO_Actions."Set") -> ("error out"=w221:errorcluster, "Stiffness Jacobian Out"=w222:T18)  [unwired: 6 out]
        n109 = Bundle By Name(cluster=T32 {"Change State"=enum."Stiffness Jacobian", "LBCB Number"=enum."LBCB1"} ("element"), "LBCB Number"=w219) -> (w225:T32)
        n110 = call "Stiffness Jacobian DAO.vi"("error in (no error)"=w221, "Stiffness Jacobian In"=w222, "LBCB Number"=w219, "Actions"=Persistant_DAO_Actions."Set") -> ("error out"=w220:errorcluster)  [unwired: 5 in, 2 out]
        n111 = Enqueue Element(queue=w232, element=w225, error in (no error)=w220) -> (queue out=w229:refnum<queue>, error out=w230:errorcluster)  [unwired: 2 out]
      }
      event #10 {
        n112 = event-data() -> ("NewVal"=w234:T11)  [unwired: 1 out]
        n113 = call "Mixed Mode Force Group Priorities DAO.vi"("Force Error Range Actions"=Persistant_DAO_Actions."Set" ("Actions"), "LBCB Number"=w235, "Force Group Priorities In"=w234, "error in (no error)"=w238) -> ("error out"=w237:errorcluster)  [unwired: 9 in, 2 out]
        n114 = Bundle By Name(cluster=T32 {"Change State"=enum."Mixed Mode", "LBCB Number"=enum."LBCB1"} ("element"), "LBCB Number"=w235) -> (w236:T32)
        n115 = Enqueue Element(queue=w244, element=w236, error in (no error)=w237) -> (queue out=w241:refnum<queue>, error out=w242:errorcluster)  [unwired: 2 out]
      }
      event #11 {
        n116 = event-data() -> ("NewVal"=w246:T14)  [unwired: 1 out]
        n117 = call "Stiffness Limits DAO.vi"("Cartesian Force Limit Actions"=Persistant_DAO_Actions."Set" ("Actions"), "ID"=w247, "Stiffness Limit In"=w246, "error in (no error)"=w250) -> ("error out"=w249:errorcluster)  [unwired: 9 in, 2 out]
        n118 = Bundle By Name(cluster=T32 {"Change State"=enum."Stiffness Jacobian", "LBCB Number"=enum."LBCB1"} ("element"), "LBCB Number"=w247) -> (w248:T32)
        n119 = Enqueue Element(queue=w256, element=w248, error in (no error)=w249) -> (queue out=w253:refnum<queue>, error out=w254:errorcluster)  [unwired: 2 out]
      }
      event #12 {
        n120 = event-data() -> ("NewVal"=w258:T13)  [unwired: 1 out]
        n121 = call "Force Control Parameters DAO.vi"("error in (no error)"=w262, "Force Control Parameters In"=w258, "DAO Actions"=Persistant_DAO_Actions."Set" ("Actions")) -> ("error out"=w261:errorcluster)  [unwired: 6 in, 2 out]
        n122 = Bundle By Name(cluster=T32 {"Change State"=enum."Mixed Mode", "LBCB Number"=enum."LBCB1"} ("element"), "LBCB Number"=w259) -> (w260:T32)
        n123 = Enqueue Element(queue=w268, element=w260, error in (no error)=w261) -> (queue out=w265:refnum<queue>, error out=w266:errorcluster)  [unwired: 2 out]
      }
      event #13 {
        n124 = event-data() -> ("NewVal"=w270:T12)  [unwired: 1 out]
        n125 = call "Mixed Mode Max Increment DAO.vi"("Max Increment Actions"=Persistant_DAO_Actions."Set" ("Actions"), "Max Increment In"=w270, "LBCB Number"=w271, "error in (no error)"=w274) -> ("error out"=w273:errorcluster)  [unwired: 9 in, 2 out]
        n126 = Bundle By Name(cluster=T32 {"Change State"=enum."Mixed Mode", "LBCB Number"=enum."LBCB1"} ("element"), "LBCB Number"=w271) -> (w272:T32)
        n127 = Enqueue Element(queue=w280, element=w272, error in (no error)=w273) -> (queue out=w277:refnum<queue>, error out=w278:errorcluster)  [unwired: 2 out]
      }
      event #14 {
        n128 = event-data() -> ("NewVal"=w282:T12)  [unwired: 1 out]
        n129 = call "Mixed Mode Jacobian Gain DAO.vi"("Jacobian Gain Actions"=Persistant_DAO_Actions."Set" ("Actions"), "Jacobian Gain In"=w282, "LBCB Number"=w283, "error in (no error)"=w286) -> ("error out"=w285:errorcluster)  [unwired: 9 in, 2 out]
        n130 = Bundle By Name(cluster=T32 {"Change State"=enum."Mixed Mode", "LBCB Number"=enum."LBCB1"} ("element"), "LBCB Number"=w283) -> (w284:T32)
        n131 = Enqueue Element(queue=w292, element=w284, error in (no error)=w285) -> (queue out=w289:refnum<queue>, error out=w290:errorcluster)  [unwired: 2 out]
      }
      event #15 {
        n132 = event-data() -> ("NewVal"=w294:T11)  [unwired: 1 out]
        n133 = call "Mixed Mode Force Error Range DAO.vi"("Force Error Range Actions"=Persistant_DAO_Actions."Set" ("Actions"), "Force Error Range In"=w294, "LBCB Number"=w295, "error in (no error)"=w298) -> ("error out"=w297:errorcluster)  [unwired: 9 in, 2 out]
        n134 = Bundle By Name(cluster=T32 {"Change State"=enum."Mixed Mode", "LBCB Number"=enum."LBCB1"} ("element"), "LBCB Number"=w295) -> (w296:T32)
        n135 = Enqueue Element(queue=w304, element=w296, error in (no error)=w297) -> (queue out=w301:refnum<queue>, error out=w302:errorcluster)  [unwired: 2 out]
      }
      event #16 {
        n136 = event-data() -> ("NewVal"=w308:T21)  [unwired: 1 out]
        n137 = call "Auto Balance Error Tolerance DAO.vi"("Auto Balance Increment Actions"=Persistant_DAO_Actions."Set" ("Actions"), "Auto Balance Error In"=w308, "LBCB Number"=w309, "error in (no error)"=w310) -> ("error out"=w306:errorcluster)  [unwired: 9 in, 2 out]
      }
      event #17 {
        n138 = event-data() -> ("NewVal"=w316:T22)  [unwired: 1 out]
        n139 = call "Autobalance Control DAO.vi"("error in (no error)"=w317, "Autobalance Control In"=w316, "Persistent DAO Actions"=Persistant_DAO_Actions."Set" ("Actions")) -> ("error out"=w315:errorcluster)  [unwired: 6 in, 2 out]
      }
    }
    n140 = local write "Application Timing and Logging"(w77) -> ()
    n141 = local write "Snapshot"(w70) -> ()
    n142 = local write "Start Autobalance"(w70) -> ()
    n143 = local read "stop"() -> (w76:bool)
    n144 = call "Error Logger.vi"("error in (no error)"=w82) -> ("error out"=w81:errorcluster)  [unwired: 1 in, 9 out]
  }
  n145 = while {
    shift-right: [w338] -> _
    shift-left: AppStates."Starting OM" ("State") -> [_]
    shift-right: [w337] -> _
    shift-left: w26 -> [w333]
    shift-right: [w335] -> _
    shift-left: w26 -> [w334]
    tunnel: w1 -> [w336]
    shift-right: [w331] -> _
    shift-left: w5 -> [w332]
    tunnel: [w324] -> w24
    shift-right: [w328] -> _
    shift-left: w16 -> [w340]
    shift-right: [w325] -> _
    shift-left: w19 -> [w326]
    stop <- w324 stop-if-true
    # "Master Loop"
    n146 = call "App Status Globals.vi"("App Status Actions"=App_Status_Actions."Get Status", "error in (no error)"=w340) -> ("App Status Out"=w322:T52, "error out"=w327:errorcluster)  [unwired: 4 in, 8 out]
    n147 = Unbundle By Name(w322) -> ("App State"=w338:T6)
    "State" <- w338
    n148 = case shown="\"Setting Up DAQ Channels\"" w338 {
      tunnel: [u32 100 ("millisecond multiple") u32 100 ("millisecond multiple") u32 100 ("millisecond multiple") u32 100 ("millisecond multiple") w510 u32 100 ("millisecond multiple") u32 45 ("millisecond multiple") u32 100 ("millisecond multiple")] -> w339
      tunnel: [w348 w385 w411 w445 w505 w519 w530 w713] -> w337
      tunnel: w336 -> [w342 w376 _ _ _ _ w532 _]
      tunnel: [w347 w384 w410 w444 w504 w518 w542 w712] -> w335
      tunnel: w334 -> [w347 w384 w410 w444 w504 w518 w541 w712]
      tunnel: w333 -> [w348 w385 w411 w445 w505 w519 w540 w713]
      tunnel: w332 -> [w346 w383 w412 w430 w506 w524 w539 w711]
      tunnel: [w346 w383 w412 w430 w506 w527 w537 w702] -> w331
      tunnel: [_ _ _ _ _ _ _ TRUE] -> w330
      tunnel: [w345 w380 w405 w419 w503 w521 w534 w703] -> w329
      tunnel: w327 -> [w345 w381 w403 w432 w501 w523 w536 w701]
      tunnel: w326 -> [w344 w379 w408 w431 w502 w525 w533 w708]
      tunnel: [w344 w379 w408 w431 w502 w525 w533 w706] -> w325
      tunnel: T26 {"Command"=enum."Start", "LBCB Number"=enum."LBCB1"} ("notification") -> [_ _ _ _ _ _ _ w698]
      frame #0 {
        (unwired) AppStates."Initializing Displays" ("State")
        n149 = call "Load Previous Command.vi"("Number of LBCBs"=w342) -> ()  [unwired: 3 in]
        n150 = call "App Status Globals.vi"("App Status Actions"=App_Status_Actions."Set App State") -> ()  [unwired: 5 in, 10 out]
        n151 = property on="Fake" class="Bool (strict)"("Visible"=FALSE) -> ()  [unwired: 2 in, 2 out]
      }
      frame #1 {
        w353 = Persistant_DAO_Actions."Get" ("DAO Actions")
        w360 = LBCB_Number."LBCB1" ("LBCB Number")
        w368 = 2.0 ("y")
        w372 = T35."Disabled and Grayed Out" ("Disabled")
        w363 = TRUE
        w391 = FALSE
        n152 = call "Working Directory.vi"() -> ("Path"=w386:path)  [unwired: 1 out]
        n153 = local write "L1 Displacement Limit"(w363) -> ()
        n154 = local write "L2 Displacement Limit"(w363) -> ()
        n155 = local write "L1 Force Limit"(w363) -> ()
        n156 = local write "L2 Force Limit"(w363) -> ()
        n157 = local write "L2 Auto Balance"(w363) -> ()
        n158 = local write "L1 Auto Balance"(w363) -> ()
        n159 = call "Actuator Disp Boundary DAO.vi"("Actions"=Persistant_DAO_Actions."Get") -> ("Limit Boundary Parameters Out"=w370:T53)  [unwired: 8 in, 2 out]
        n160 = Unbundle By Name(w370) -> ("Lower"=w369:dbl, "Upper"=w367:dbl)
        n161 = call "NoArgumentsLauncher.vi"("Application Launcher Actions"=Launcher_Actions."Init") -> ()  [unwired: 2 in, 9 out]
        n162 = property on="Raw Data" class="Arr (strict)"("Label.FontSize"=u32 18 ("Label.Font:Size")) -> ()  [unwired: 2 in, 2 out]
        n163 = local write "L1 Control"(w391) -> ()
        n164 = Build Path(base path=w386, name or relative path="image") -> (appended path=w389:path)
        n165 = local write "LBCB Number Button"(w391) -> ()
        n166 = local write "Cartesian Type"(w391) -> ()
        n167 = local write "L2 Control"(w391) -> ()
        n168 = local write "stop"(w391) -> ()
        n169 = property on="Start Autobalance" class="Bool (strict)"("DisabledEnum"=T35."Enabled" ("Disabled")) -> ()  [unwired: 2 in, 2 out]
        n170 = Build Path(base path=w389, name or relative path="UILogoCL1c_mdf.bmp") -> (appended path=w387:path)
        n171 = call "Log Filenames List.vi"("Log Filename Actions"=Log_Filename_Actions."Init") -> ()  [unwired: 3 in, 8 out]
        n172 = Equal?(x=Number_Of_LBCBs."2", y=w376) -> (x = y?=w377:bool)
        n173 = Divide(x=w369, y=w368) -> (x/y=w366:dbl)
        n174 = property on="L2 Control" class="Bool (strict)"("Disabled"=w372) -> ()  [unwired: 2 in, 2 out]
        n175 = Divide(x=w367, y=w368) -> (x/y=w365:dbl)
        n176 = Select(t=T35."Enabled" ("Disabled"), s=w377, f=T35."Disabled") -> (s? t:f=w378:T35)
        n177 = property on="L1 Control" class="Bool (strict)"("Disabled"=w372) -> ()  [unwired: 2 in, 2 out]
        n178 = call "Load Cache.vi"() -> ()  [unwired: 1 out]
        n179 = property on="LBCB Number Button" class="Bool (strict)"("Disabled"=w378) -> ()  [unwired: 2 in, 2 out]
        n180 = call <vilib>:"Read BMP File.vi"("error in (no error)"=w381, "path to BMP file"=w387) -> ("error out"=w380:errorcluster, "image data"=w400:T54)  [unwired: 8 out]
        n181 = property on="Actuator X1" class="Slide (strict)"("DisabledEnum"=w372, "Scale.Minimum"=w369, "Scale.Maximum"=w367) -> ()  [unwired: 2 in, 2 out]
        n182 = property on="Actuator X2" class="Slide (strict)"("DisabledEnum"=w372, "Scale.Minimum"=w369, "Scale.Maximum"=w367) -> ()  [unwired: 2 in, 2 out]
        n183 = property on="Actuator Y1" class="Slide (strict)"("DisabledEnum"=w372, "Scale.Minimum"=w366, "Scale.Maximum"=w365) -> ()  [unwired: 2 in, 2 out]
        n184 = property on="Actuator Z1" class="Slide (strict)"("DisabledEnum"=w372, "Scale.Minimum"=w366, "Scale.Maximum"=w365) -> ()  [unwired: 2 in, 2 out]
        n185 = property on="Actuator Z2" class="Slide (strict)"("DisabledEnum"=w372, "Scale.Minimum"=w366, "Scale.Maximum"=w365) -> ()  [unwired: 2 in, 2 out]
        n186 = property on="Actuator Z3" class="Slide (strict)"("DisabledEnum"=w372, "Scale.Minimum"=w366, "Scale.Maximum"=w365) -> ()  [unwired: 2 in, 2 out]
        n187 = call "ConfigPath.vi"("Config Path Actions"=ConfigPathActions."Init") -> ()  [unwired: 2 in, 9 out]
        n188 = call <vilib>:"Draw Flattened Pixmap.vi"("image data"=w400) -> ("new picture"=→"Logo":picture)  [unwired: 1 in, 7 out]
        n189 = call "Autobalance Control DAO.vi"("Persistent DAO Actions"=w353) -> ("Autobalance Control Out"=w359:T22)  [unwired: 8 in, 2 out]
        n190 = call "Stiffness Limits DAO.vi"("Cartesian Force Limit Actions"=w353, "ID"=w360) -> ("Stiffness Limit Out"=w354:T44)  [unwired: 11 in, 2 out]
        n191 = call "Auto Balance Error Tolerance DAO.vi"("Auto Balance Increment Actions"=w353, "LBCB Number"=w360) -> ("Auto Balance Error Out"=w355:T21)  [unwired: 11 in, 2 out]
        n192 = call "Mixed Mode Force Group Priorities DAO.vi"("Force Error Range Actions"=w353, "LBCB Number"=w360) -> ("Force Group Priorities Out"=w351:T11)  [unwired: 11 in, 2 out]
        n193 = call "Mixed Mode Force Error Range DAO.vi"("Force Error Range Actions"=w353, "LBCB Number"=w360) -> ("Force Error Range Out"=w357:T12)  [unwired: 11 in, 2 out]
        n194 = call "Mixed Mode Max Increment DAO.vi"("Max Increment Actions"=w353, "LBCB Number"=w360) -> ("Max Increment Out"=w356:T12)  [unwired: 11 in, 2 out]
        n195 = call "Mixed Mode Jacobian Gain DAO.vi"("Jacobian Gain Actions"=w353, "LBCB Number"=w360) -> ("Jacobian Gain Out"=w358:T12)  [unwired: 11 in, 2 out]
        n196 = call "Force Control Parameters DAO.vi"("DAO Actions"=w353) -> ("Force Control Parameters Out"=w352:T13)  [unwired: 8 in, 2 out]
        n197 = call "FaultsList.vi"("Limits List Actions"=Faults_List_Actions."Init") -> ()  [unwired: 2 in, 9 out]
        n198 = local write "Force Control Parameters"(w352) -> ()
        n199 = local write "Auto Balance Error Window"(w355) -> ()
        n200 = local write "Auto Balance Control"(w359) -> ()
        n201 = local write "Force Group Priorities"(w351) -> ()
        n202 = local write "Stiffness Limit"(w354) -> ()
        n203 = local write "Max Increment"(w356) -> ()
        n204 = local write "Jacobian Gain"(w358) -> ()
        n205 = local write "Force Error Range"(w357) -> ()
        n206 = call "PID Controls DAO.vi"("LBCB Number"=w360, "Actions"=DAO_Actions."Get") -> ("PID Control  Out"=w362:T4)  [unwired: 8 in, 1 out]
        n207 = call "App Status Globals.vi"("App Status Actions"=App_Status_Actions."Set App State", "App State"=AppStates."Setting up Archiving" ("State")) -> ()  [unwired: 4 in, 10 out]
        n208 = local write "PID Control"(w362) -> ()
      }
      frame #2 {
        w404 = DAO_Actions."Init" ("DAO Actions")
        n209 = call "App Status Globals.vi"("App Status Actions"=App_Status_Actions."Set App State", "App State"=AppStates."Setting Up DAQ Channels" ("State")) -> ()  [unwired: 4 in, 10 out]
        n210 = call "Assemble Archive Headers.vi"("error in"=w403) -> ("External Sensor Names"=w402:string[], "error out"=w401:errorcluster)
        n211 = call "Individual Cartesian Measurements.vi"("DAO Actions"=w404) -> ()  [unwired: 7 in, 4 out]
        n212 = call "MM Multi DOF Status DAO.vi"("Actions"=w404) -> ()  [unwired: 9 in, 2 out]
        n213 = local write "External Sensor Names"(w402) -> ()
        n214 = call "NoArgumentsLauncher.vi"("error in (no error)"=w401, "Application"=NoPanelAppTypes."Data Archiving", "Application Launcher Actions"=Launcher_Actions."Launch") -> ("error out"=w405:errorcluster)  [unwired: 8 out]
      }
      frame #3 {
        w439 = Cartesian_Measurment_Actions."Init" ("Measurement Actions")
        # "Assume both LBCBs are \nthe same size"
        n215 = call "ConsolidatedDAQChannelNames.vi"() -> ("Consolidated Task Names"=w435:string)  [unwired: 5 out]
        n216 = call "App Parameters DAO.vi"("Actions"=Persistant_DAO_Actions."Get") -> ("Application Timing and Logging Out"=w416:T7)  [unwired: 3 in, 7 out]
        n217 = local read "Fake"() -> (w429:bool)
        n218 = call "Daq Receive.vi"("Daq Actions"=Daq_Actions."Init", "error in (no error)"=w432, "Fake"=w429) -> ("error out"=w436:errorcluster)  [unwired: 7 out]
        n219 = case shown="Error" w436 {
          selector: w436 -> [w472 w480]
          tunnel: [w469 w480] -> w438
          tunnel: [w471 AppStates."Stopping OM" ("State")] -> w437
          tunnel: w435 -> [_ w483]
          tunnel: w429 -> [w467 _]
          frame #0 {
            n220 = call "Daq Send.vi"("Fake"=w467, "error in (no error)"=w472, "LBCB Select"=LBCB_Number."LBCB2", "Daq Actions"=Daq_Actions."Init") -> ("error out"=w470:errorcluster)  [unwired: 1 in, 6 out]
            n221 = case shown="No Error" w470 {
              selector: w470 -> [w474 w477]
              tunnel: [AppStates."Start DAQ" ("State") AppStates."Stopping OM" ("State")] -> w471
              tunnel: [w474 w477] -> w469
              frame #0 {
              }
              frame #1 {
                n222 = One Button Dialog(message="DAQ Send\nChannels\nare not \nconfigured\ncorrectly") -> ()  [unwired: 2 out]
              }
            }
          }
          frame #1 {
            n223 = Concatenate Strings("DAQ Receive Channels\nnot configured correctly:\n  " ("string"), w483) -> (w481:string)
            n224 = One Button Dialog(message=w481) -> ()  [unwired: 2 out]
          }
        }
        n225 = Unbundle By Name(w416) -> ("Logging Directory"=w417:path)
        n226 = call <vilib>:"Clear Errors.vi"("error in (no error)"=w438) -> ("error out"=w433:errorcluster)  [unwired: 6 out]
        n227 = call "App Status Globals.vi"("App Status Actions"=App_Status_Actions."Set App State", "App State"=w437, "error in (no error)"=w433) -> ("error out"=w434:errorcluster)  [unwired: 3 in, 9 out]
        n228 = call "LBCB Settings DAO.vi"("error in (no error)"=w434, "LBCB Number"=LBCB_Number."LBCB1", "Actions"=Persistant_DAO_Actions."Get") -> ("error out"=w421:errorcluster, "LBCB Setting Out"=w442:T37)  [unwired: 2 in, 5 out]
        n229 = call "Log Filenames List.vi"("error in (no error)"=w421, "LogFile Type"=LogFileType."DLL  Errors", "Log Filename Actions"=Log_Filename_Actions."Get Filename") -> ("error out"=w425:errorcluster, "Filename"=w424:path)  [unwired: 1 in, 6 out]
        n230 = Strip Path(path=w424) -> (stripped path=w422:path)  [unwired: 1 out]
        n231 = call <vilib>:"Check if File or Folder Exists.vi"("error in (no error)"=w425, "path"=w422) -> ("error out"=w426:errorcluster, "file or folder exists?"=w427:bool)  [unwired: 8 out]
        n232 = Unbundle By Name(w442) -> ("Size"=w420:T38)
        n233 = case shown="True" w427 {
          tunnel: w426 -> [w485 w492]
          tunnel: w424 -> [w491 w500]
          tunnel: [w484 w494] -> w423
          tunnel: w420 -> [_ w497]
          frame #0 {
            n234 = Path To String(path=w491) -> (string=w490:string)
            n235 = Concatenate Strings(w490, " does not exist" ("string")) -> (w488:string)
            n236 = call "App Status Globals.vi"("App Status Actions"=App_Status_Actions."Set App State", "App State"=AppStates."Stopping OM", "error in (no error)"=w485) -> ("error out"=w484:errorcluster)  [unwired: 3 in, 9 out]
            n237 = One Button Dialog(message=w488) -> ()  [unwired: 2 out]
          }
          frame #1 {
            n238 = Path To String(path=w500) -> (string=w499:string)
            n239 = call "LBCB_Conversions.vi"("Size"=w497, "error in (no error)"=w492, "Error Log \nFilename"=w499, "Conversion Type"=LBCB_Conversions_Actions."Init") -> ("error out"=w495:errorcluster)  [unwired: 4 in, 3 out]
            n240 = call "NoArgumentsLauncher.vi"("error in (no error)"=w495, "Application"=NoPanelAppTypes."Control Loops", "Application Launcher Actions"=Launcher_Actions."Launch") -> ("error out"=w494:errorcluster)  [unwired: 8 out]
          }
        }
        n241 = call "Actuator Data Set.vi"("error in (no error)"=w423, "Measurement Actions"=Actuator_Measurment_Actions."Init") -> ("error out"=w450:errorcluster)  [unwired: 3 in, 6 out]
        n242 = call "Cartesian Data Set.vi"("Measurement Actions"=w439, "error in (no error)"=w450) -> ("error out"=w449:errorcluster)  [unwired: 4 in, 9 out]
        n243 = call "External Sensors Data Set.vi"("Measurement Actions"=w439, "error in (no error)"=w449) -> ("error out"=w428:errorcluster)  [unwired: 9 in, 4 out]
        n244 = call "Save Archive Headers.vi"("error in (no error)"=w428) -> ("error out"=w418:errorcluster)  [unwired: 10 out]
        n245 = case shown="Error" w418 {
          selector: w418 -> [w453 w460]
          tunnel: [w453 w455] -> w419
          tunnel: w417 -> [_ w454]
          frame #0 {
          }
          frame #1 {
            n246 = flat-sequence {
              tunnel: w460 -> [w466]
              tunnel: [w466] -> w459
              tunnel: w454 -> [w465]
              frame #0 {
                n247 = Path To String(path=w465) -> (string=w464:string)
                n248 = Concatenate Strings("Log folder \"" ("string"), w464, "\" cannot be written to.  Use OM setup to fix this." ("string")) -> (w463:string)
                n249 = One Button Dialog(message=w463) -> ()  [unwired: 1 in, 1 out]
              }
            }
            n250 = call "App Status Globals.vi"("App Status Actions"=App_Status_Actions."Set App State", "App State"=AppStates."Stopping OM", "error in (no error)"=w459) -> ("error out"=w458:errorcluster)  [unwired: 3 in, 9 out]
            n251 = call <vilib>:"Clear Errors.vi"("error in (no error)"=w458) -> ("error out"=w455:errorcluster)  [unwired: 6 in]
          }
        }
      }
      frame #4 {
        n252 = call "App Status Globals.vi"("App Status Actions"=App_Status_Actions."DAQ Started", "Status\nSetting"=TRUE ("Status\nSetting"), "error in (no error)"=w501) -> ("error out"=w507:errorcluster)  [unwired: 3 in, 9 out]
        n253 = call "App Status Globals.vi"("App Status Actions"=App_Status_Actions."Get Status", "error in (no error)"=w507) -> ("App Status Out"=w512:T52, "error out"=w503:errorcluster)  [unwired: 4 in, 8 out]
        n254 = Unbundle By Name(w512) -> ("Data Acquisition"=w511:bool)
        n255 = case shown="True" w511 {
          tunnel: [u32 100 ("millisecond multiple") u32 200 ("millisecond multiple")] -> w510
          frame #0 {
          }
          frame #1 {
            n256 = call "App Status Globals.vi"("App Status Actions"=App_Status_Actions."Set App State", "App State"=AppStates."Controlling LBCBs" ("State")) -> ()  [unwired: 4 in, 10 out]
          }
        }
      }
      frame #5 {
        # "Assume both LBCBs are \nthe same size"
        # "Assumes that the external channel names are last"
        n257 = Enqueue Element(queue=w524, element=T32 {"Change State"=enum."Start DAQ", "LBCB Number"=enum."LBCB1"}, error in (no error)=w523) -> (queue out=w527:refnum<queue>, error out=w522:errorcluster)  [unwired: 2 out]
        n258 = call "App Status Globals.vi"("App Status Actions"=App_Status_Actions."Set App State", "App State"=AppStates."DAQ Starting", "error in (no error)"=w522) -> ("error out"=w521:errorcluster)  [unwired: 3 in, 9 out]
      }
      frame #6 {
        n259 = local read "Start AB Selected"() -> (w531:bool)
        n260 = case shown="\"Start Selected\"" w540 {
          selector: w540 -> [_ _ _ _ w583 w596 w609]
          tunnel: [w549 w560 Lbcb_Control_Loop_States."Control Loop Initialized" ("t") Lbcb_Control_Loop_States."Autobalancing" ("f") w587 w600 w610] -> w530
          tunnel: w539 -> [w547 w558 w569 w580 w592 w605 w614]
          tunnel: [w547 w558 w567 w578 w592 w605 w614] -> w538
          tunnel: w536 -> [w544 w554 w564 w571 w586 w599 w607]
          tunnel: [w546 w557 w565 w576 w585 w598 w606] -> w535
          tunnel: w531 -> [w545 _ _ _ w582 w597 _]
          frame #0 {
            n261 = Select(t=Lbcb_Control_Loop_States."Start Selected" ("LBCB State"), s=w545, f=Lbcb_Control_Loop_States."Idle") -> (s? t:f=w549:T3)
            n262 = call "App Status Globals.vi"("App Status Actions"=App_Status_Actions."Set LBCB State", "LBCB Number"=LBCB_Number."LBCB1", "error in (no error)"=w544, "LBCB State"=w549) -> ("error out"=w546:errorcluster)  [unwired: 3 in, 8 out]
          }
          frame #1 {
            n263 = call "LBCB Initialization & Autobalancing.vi"("Selected LBCB"=LBCB_Number."LBCB1", "error in (no error)"=w554) -> ("Use Previous\nCommand"=w555:bool, "error out"=w553:errorcluster)  [unwired: 7 out]
            n264 = Select(t=Lbcb_Control_Loop_States."Load Last Command" ("LBCB State"), s=w555, f=Lbcb_Control_Loop_States."Start Autobalancing") -> (s? t:f=w560:T3)
            n265 = call "App Status Globals.vi"("App Status Actions"=App_Status_Actions."Set LBCB State", "LBCB Number"=LBCB_Number."LBCB1", "error in (no error)"=w553, "LBCB State"=w560) -> ("error out"=w557:errorcluster)  [unwired: 3 in, 8 out]
          }
          frame #2 {
            n266 = Enqueue Element(queue=w569, element=T32 {"Change State"=enum."Set Command", "LBCB Number"=enum."LBCB1"}, error in (no error)=w564) -> (queue out=w567:refnum<queue>, error out=w565:errorcluster)  [unwired: 2 out]
          }
          frame #3 {
            n267 = call "App Status Globals.vi"("App Status Actions"=App_Status_Actions."Autobalanced", "LBCB Number"=LBCB_Number."LBCB1", "Status\nSetting"=FALSE ("Status\nSetting"), "error in (no error)"=w571) -> ("error out"=w570:errorcluster)  [unwired: 3 in, 8 out]
            n268 = Enqueue Element(queue=w580, element=T32 {"Change State"=enum."Reset Auto-Balance", "LBCB Number"=enum."LBCB1"}, error in (no error)=w570) -> (queue out=w578:refnum<queue>, error out=w576:errorcluster)  [unwired: 2 out]
            n269 = property on="L1 Control" class="Bool (strict)"("Disabled"=T35."Disabled and Grayed Out") -> ()  [unwired: 2 in, 2 out]
          }
          frame #4 {
            n270 = call "App Status Globals.vi"("App Status Actions"=App_Status_Actions."Get Status", "error in (no error)"=w586) -> ("App Status Out"=w590:T52, "error out"=w585:errorcluster)  [unwired: 4 in, 8 out]
            n271 = Unbundle By Name(w590) -> ("Autobalance L1"=w589:bool)
            n272 = Select(t=Lbcb_Control_Loop_States."Start Selected", s=w582, f=w583) -> (s? t:f=w581:T3)
            n273 = Select(t=Lbcb_Control_Loop_States."Control Loop Initialized", s=w589, f=w581) -> (s? t:f=w587:T3)
          }
          frame #5 {
            n274 = call "App Status Globals.vi"("App Status Actions"=App_Status_Actions."Get Status", "error in (no error)"=w599) -> ("App Status Out"=w603:T52, "error out"=w598:errorcluster)  [unwired: 4 in, 8 out]
            n275 = property on="L1 Control" class="Bool (strict)"("Disabled"=T35."Enabled") -> ()  [unwired: 2 in, 2 out]
            n276 = Unbundle By Name(w603) -> ("Controlling L1"=w602:bool)
            n277 = Select(t=Lbcb_Control_Loop_States."Start Selected", s=w597, f=w596) -> (s? t:f=w595:T3)
            n278 = Select(t=Lbcb_Control_Loop_States."Control Enabled", s=w602, f=w595) -> (s? t:f=w600:T3)
          }
          frame #6 {
            n279 = call "App Status Globals.vi"("App Status Actions"=App_Status_Actions."Get Status", "error in (no error)"=w607) -> ("App Status Out"=w612:T52, "error out"=w606:errorcluster)  [unwired: 4 in, 8 out]
            n280 = Unbundle By Name(w612) -> ("Controlling L1"=w611:bool)
            n281 = Select(t=w609, s=w611, f=Lbcb_Control_Loop_States."Control Loop Initialized" ("t")) -> (s? t:f=w610:T3)
          }
        }
        n282 = case shown="\"2\"" w532 {
          tunnel: [Lbcb_Control_Loop_States."Idle" ("f") w625] -> w542
          tunnel: w541 -> [_ w626]
          tunnel: w538 -> [w617 w624]
          tunnel: [w617 w623] -> w537
          tunnel: w535 -> [w616 w622]
          tunnel: [w616 w621] -> w534
          tunnel: w531 -> [_ w620]
          tunnel: w530 -> [w615 _]
          frame #0 {
            n283 = case shown="\"Start Selected\"" w615 {
              frame #0 {
              }
              frame #1 {
                n284 = local write "Start AB Selected"(FALSE ("Start AB Selected")) -> ()
              }
            }
          }
          frame #1 {
            n285 = case shown="\"Control Enabled\"" w626 {
              selector: w626 -> [_ _ _ _ w665 w679 w689]
              tunnel: [w630 w641 Lbcb_Control_Loop_States."Control Loop Initialized" ("t") Lbcb_Control_Loop_States."Autobalancing" ("f") w670 w682 w691] -> w625
              tunnel: w624 -> [w629 w640 w651 w663 w669 w681 w690]
              tunnel: [w629 w640 w649 w661 w669 w681 w690] -> w623
              tunnel: w622 -> [w628 w638 w646 w653 w668 w680 w687]
              tunnel: [w628 w637 w647 w659 w668 w680 w687] -> w621
              tunnel: w620 -> [w627 _ _ _ w666 w677 _]
              frame #0 {
                n286 = Select(t=Lbcb_Control_Loop_States."Start Selected" ("LBCB State"), s=w627, f=Lbcb_Control_Loop_States."Idle") -> (s? t:f=w630:T3)
                n287 = call "App Status Globals.vi"("App Status Actions"=App_Status_Actions."Set LBCB State", "LBCB Number"=LBCB_Number."LBCB2", "LBCB State"=w630) -> ()  [unwired: 4 in, 9 out]
              }
              frame #1 {
                n288 = local write "Start AB Selected"(FALSE ("Start Autobalance")) -> ()
                n289 = call "LBCB Initialization & Autobalancing.vi"("Selected LBCB"=LBCB_Number."LBCB2", "error in (no error)"=w638) -> ("Use Previous\nCommand"=w636:bool, "error out"=w637:errorcluster)  [unwired: 1 in, 6 out]
                n290 = Select(t=Lbcb_Control_Loop_States."Load Last Command" ("LBCB State"), s=w636, f=Lbcb_Control_Loop_States."Start Autobalancing") -> (s? t:f=w641:T3)
                n291 = call "App Status Globals.vi"("App Status Actions"=App_Status_Actions."Set LBCB State", "LBCB Number"=LBCB_Number."LBCB2", "LBCB State"=w641) -> ()  [unwired: 4 in, 9 out]
              }
              frame #2 {
                n292 = Enqueue Element(queue=w651, element=T32 {"Change State"=enum."Set Command", "LBCB Number"=enum."LBCB2"}, error in (no error)=w646) -> (queue out=w649:refnum<queue>, error out=w647:errorcluster)  [unwired: 2 out]
              }
              frame #3 {
                n293 = call "App Status Globals.vi"("App Status Actions"=App_Status_Actions."Autobalanced", "LBCB Number"=LBCB_Number."LBCB2", "Status\nSetting"=FALSE ("Status\nSetting"), "error in (no error)"=w653) -> ("error out"=w652:errorcluster)  [unwired: 3 in, 8 out]
                n294 = local write "Start AB Selected"(FALSE ("Start AB Selected")) -> ()
                n295 = Enqueue Element(queue=w663, element=T32 {"Change State"=enum."Reset Auto-Balance", "LBCB Number"=enum."LBCB2"}, error in (no error)=w652) -> (queue out=w661:refnum<queue>, error out=w659:errorcluster)  [unwired: 2 out]
                n296 = property on="L2 Control" class="Bool (strict)"("DisabledEnum"=T35."Disabled and Grayed Out" ("Disabled")) -> ()  [unwired: 2 in, 2 out]
              }
              frame #4 {
                n297 = call "App Status Globals.vi"("App Status Actions"=App_Status_Actions."Get Status") -> ("App Status Out"=w672:T52)  [unwired: 5 in, 9 out]
                n298 = Unbundle By Name(w672) -> ("Autobalance L2"=w673:bool)
                n299 = Select(t=Lbcb_Control_Loop_States."Start Selected", s=w666, f=w665) -> (s? t:f=w664:T3)
                n300 = Select(t=Lbcb_Control_Loop_States."Control Loop Initialized", s=w673, f=w664) -> (s? t:f=w670:T3)
              }
              frame #5 {
                n301 = call "App Status Globals.vi"("App Status Actions"=App_Status_Actions."Get Status") -> ("App Status Out"=w684:T52)  [unwired: 5 in, 9 out]
                n302 = Unbundle By Name(w684) -> ("Controlling L2"=w685:bool)
                n303 = Select(t=Lbcb_Control_Loop_States."Start Selected", s=w677, f=w679) -> (s? t:f=w678:T3)
                n304 = property on="L2 Control" class="Bool (strict)"("Disabled"=T35."Enabled") -> ()  [unwired: 2 in, 2 out]
                n305 = Select(t=Lbcb_Control_Loop_States."Control Enabled", s=w685, f=w678) -> (s? t:f=w682:T3)
              }
              frame #6 {
                n306 = call "App Status Globals.vi"("App Status Actions"=App_Status_Actions."Get Status") -> ("App Status Out"=w693:T52)  [unwired: 5 in, 9 out]
                n307 = Unbundle By Name(w693) -> ("Controlling L2"=w694:bool)
                n308 = Select(t=w689, s=w694, f=Lbcb_Control_Loop_States."Control Loop Initialized" ("t")) -> (s? t:f=w691:T3)
              }
            }
          }
        }
      }
      frame #7 {
        n309 = property on="Fake" class="Bool (strict)"("Visible"=TRUE) -> ()  [unwired: 2 in, 2 out]
        n310 = Enqueue Element(queue=w711, element=T32 {"Change State"=enum."Stop Application", "LBCB Number"=enum."LBCB1"}, error in (no error)=w701) -> (queue out=w702:refnum<queue>, error out=w700:errorcluster)  [unwired: 2 out]
        n311 = Bundle By Name(cluster=w698, "Command"=MM_Widget_Parameter_Changes."Stop All" ("notification")) -> (w696:T26)
        n312 = Send Notification(notification=w696, notifier=w708, error in (no error)=w700) -> (notifier out=w706:refnum<notifier>, error out=w707:errorcluster)
        n313 = call "App Status Globals.vi"("App Status Actions"=App_Status_Actions."Running", "Status\nSetting"=FALSE ("Status\nSetting"), "error in (no error)"=w707) -> ("error out"=w703:errorcluster)  [unwired: 3 in, 9 out]
      }
    }
    n314 = local read "stop"() -> (w323:bool)
    n315 = Or(x=w330, y=w323) -> (x .or. y?=w324:bool)
    n316 = Wait Until Next ms Multiple(millisecond multiple=w339) -> ()  [unwired: 1 out]
    n317 = call "Error Logger.vi"("error in (no error)"=w329) -> ("error out"=w328:errorcluster)  [unwired: 1 in, 9 out]
    "LBCB 1 State" <- w333
    "LBCB 2 State" <- w334
  }
  n318 = Obtain Notifier(name (unnamed)="Mixed Mode Statuses", notification data type=T25 {"LBCB Target"=[], "MixedModeStates"=enum."Init", "LBCB Convergence"=[], "LBCB Measurements"=[]} ("Mixed Mode Status"), error in (no error)=w7) -> (notifier out=w10:refnum<notifier>, error out=w9:errorcluster)  [unwired: 1 in, 1 out]
  n319 = while {
    shift-right: [w747] -> _
    shift-left: w19 -> [w748]
    tunnel: [w725] -> w23
    shift-right: [w718] -> _
    shift-left: w7 -> [w724]
    shift-right: [w720] -> _
    shift-left: w5 -> [w721]
    stop <- w725 stop-if-true
    w738 = TRUE ("Use LBCB Selector")
    # "Statuses Loop"
    n320 = local read "Application Timing and Logging"() -> (w742:T7)
    n321 = call "Messages.vi"() -> ("Messages"=w741:string)  [unwired: 1 in, 10 out]
    n322 = Unbundle By Name(w742) -> ("Monitor Loop.Interval"=w746:dbl)
    n323 = local write "Messages"(w741) -> ()
    n324 = Multiply(x=w746, y=1000.0) -> (x*y=w744:dbl)
    n325 = Wait on Notification(notifier=w748, timeout in ms (-1)=w744, error in (no error)=w724) -> (notifier out=w747:refnum<notifier>, notification=w743:T26, error out=w719:errorcluster)  [unwired: 2 out]
    n326 = Unbundle By Name(w743) -> ("Command"=w723:T27, "LBCB Number"=w722:enum16{"LBCB1", "LBCB2"})
    n327 = case shown="\"Cartesian Type Changed\"" w723 {
      tunnel: [_ w760 _ _ _] -> w725
      tunnel: w722 -> [_ _ w769 w776 _]
      tunnel: w721 -> [w751 w759 w775 w782 w784]
      tunnel: [w751 w758 w773 w780 w784] -> w720
      tunnel: w719 -> [w750 w757 w774 w781 w783]
      tunnel: [w750 w756 w772 w779 w783] -> w717
      frame #0 {
        n328 = call "App Status Globals.vi"("App Status Actions"=App_Status_Actions."Get Status") -> ("App Status Out"=w754:T52)  [unwired: 5 in, 9 out]
        n329 = Unbundle By Name(w754) -> ("Cartesian Type"=w753:bool)
        n330 = local write "Cartesian Type"(w753) -> ()
      }
      frame #1 {
        w763 = FALSE ("Status\nSetting")
        w760 = TRUE ("stop")
        n331 = local write "all stopped"(w763) -> ()
        n332 = local write "stop"(w760) -> ()
        n333 = call "App Status Globals.vi"("App Status Actions"=App_Status_Actions."Set App State", "App State"=AppStates."Stopping OM" ("State")) -> ("error out"=w767:errorcluster)  [unwired: 4 in, 9 out]
        n334 = Wait Until Next ms Multiple(millisecond multiple=u32 100) -> ()  [unwired: 1 out]
        n335 = call "App Status Globals.vi"("App Status Actions"=App_Status_Actions."Running", "Status\nSetting"=w763, "error in (no error)"=w767) -> ("error out"=w761:errorcluster)  [unwired: 3 in, 9 out]
        n336 = Enqueue Element(queue=w759, element=T32 {"Change State"=enum."Stop Application", "LBCB Number"=enum."LBCB1"}, error in (no error)=w757) -> (queue out=w758:refnum<queue>, error out=w756:errorcluster)  [unwired: 1 in, 1 out]
        n337 = call "App Status Globals.vi"("App Status Actions"=App_Status_Actions."Set DAQ Link", "Status\nSetting"=w763, "error in (no error)"=w761) -> ()  [unwired: 3 in, 10 out]
      }
      frame #2 {
        n338 = Bundle By Name(cluster=T32 {"Change State"=enum."Enable Control", "LBCB Number"=enum."LBCB1"} ("element"), "LBCB Number"=w769) -> (w770:T32)
        n339 = Enqueue Element(queue=w775, element=w770, error in (no error)=w774) -> (queue out=w773:refnum<queue>, error out=w772:errorcluster)  [unwired: 1 in, 1 out]
      }
      frame #3 {
        n340 = Bundle By Name(cluster=T32 {"Change State"=enum."Disable Control", "LBCB Number"=enum."LBCB1"} ("element"), "LBCB Number"=w776) -> (w777:T32)
        n341 = Enqueue Element(queue=w782, element=w777, error in (no error)=w781) -> (queue out=w780:refnum<queue>, error out=w779:errorcluster)  [unwired: 1 in, 1 out]
      }
      frame #4 {
      }
    }
    n342 = call "Fault List 2 Indicators.vi"("Use LBCB Selector"=w738, "LBCB Number"=LBCB_Number."LBCB2") -> ("Forces"=w734:bool, "Displacement"=w735:bool)  [unwired: 8 out]
    n343 = call "Fault List 2 Indicators.vi"("Use LBCB Selector"=w738, "LBCB Number"=LBCB_Number."LBCB1") -> ("Forces"=w736:bool, "Displacement"=w737:bool)  [unwired: 8 out]
    n344 = call "App Status Globals.vi"("App Status Actions"=App_Status_Actions."Get Status") -> ("App Status Out"=w732:T52)  [unwired: 5 in, 9 out]
    n345 = Not(x=w736) -> (.not. x?=w729:bool)
    n346 = Unbundle By Name(w732) -> ("Autobalance L1"=w731:bool, "Autobalance L2"=w730:bool, "Cartesian Type"=w714:bool)
    n347 = Not(x=w737) -> (.not. x?=w728:bool)
    n348 = Not(x=w734) -> (.not. x?=w726:bool)
    n349 = Not(x=w735) -> (.not. x?=w727:bool)
    n350 = local write "L1 Displacement Limit"(w728) -> ()
    n351 = local write "L2 Displacement Limit"(w727) -> ()
    n352 = local write "L1 Auto Balance"(w731) -> ()
    n353 = local write "L2 Auto Balance"(w730) -> ()
    n354 = local write "L1 Force Limit"(w729) -> ()
    n355 = local write "L2 Force Limit"(w726) -> ()
    n356 = local read "Cartesian Type"() -> (w716:bool)
    n357 = Not Equal?(x=w716, y=w714) -> (x != y?=w715:bool)
    n358 = case shown="True" w715 {
      tunnel: w714 -> [_ w749]
      frame #0 {
      }
      frame #1 {
        n359 = local write "Cartesian Type"(w749) -> ()
      }
    }
    n360 = call <vilib>:"Merge Errors.vi"("error in 3 (no error)"=w719, "error in 1 (no error)"=w717) -> ("error out"=w718:errorcluster)  [unwired: 5 in]
  }
  n361 = while {
    shift-right: [w786] -> _
    shift-left: w9 -> [w788]
    shift-right: [w787] -> _
    shift-left: w10 -> [w789]
    tunnel: [w785] -> w8
    stop <- w785 stop-if-true
    n362 = local read "LBCB Number Button"() -> (w798:bool)
    n363 = local read "Cartesian Type"() -> (w794:bool)
    n364 = local read "Application Timing and Logging"() -> (w791:T7)
    n365 = Unbundle By Name(w791) -> ("Monitor Loop.Interval"=w792:dbl)
    n366 = Select(t=LBCB_Number."LBCB2", s=w798, f=LBCB_Number."LBCB1" ("LBCB Number")) -> (s? t:f=w799:T5)
    n367 = local read "Monitor Panel"() -> (w795:T9)
    n368 = Multiply(x=w792, y=1000.0) -> (x*y=w790:dbl)
    n369 = local read "stop"() -> (w785:bool)
    n370 = case shown="\"Displacements  Forces\"" w795 {
      tunnel: w799 -> [w806 w818 w841 _]
      tunnel: w794 -> [_ w836 w839 _]
      tunnel: w798 -> [_ _ _ w872]
      tunnel: w790 -> [w802 w817 w840 w867]
      tunnel: w789 -> [w801 w816 w847 w866]
      tunnel: w788 -> [w800 w815 w846 w865]
      tunnel: [w801 w816 w845 w866] -> w787
      tunnel: [w800 w815 w844 w865] -> w786
      frame #0 {
        n371 = local read "External Sensor Names"() -> (w804:string[])
        n372 = call "Actuator Data Set.vi"("Selected LBCB"=w806, "Measurement Actions"=Actuator_Measurment_Actions."Get") -> ("Volts Out"=w807:T56)  [unwired: 3 in, 6 out]
        n373 = call "Generate External Sensors Table.vi"("External Sensor Names"=w804, "Use Volts"=TRUE) -> ("External Sensors"=w803:cluster{"Name":string, "Value":dbl}[])  [unwired: 1 in, 8 out]
        n374 = Wait Until Next ms Multiple(millisecond multiple=w802) -> ()  [unwired: 1 out]
        n375 = Unbundle By Name(w807) -> ("Commands"=w813:dbl[], "LVDTs"=w812:dbl[], "Load Cells"=w811:dbl[], "Servo"=w810:dbl[])
        n376 = local write "External Sensors Volts"(w803) -> ()
        n377 = Build Array(w813, w812, w811, w810) -> (w809:dbl[][])
        n378 = Transpose 2D Array(2D array=w809) -> (transposed array=→"Raw Data":dbl[][])
      }
      frame #1 {
        n379 = local read "External Sensor Names"() -> (w834:string[])
        n380 = Wait Until Next ms Multiple(millisecond multiple=w817) -> ()  [unwired: 1 out]
        n381 = call "Generate External Sensors Table.vi"("External Sensor Names"=w834, "WithOffset"=w836) -> ("External Sensors"=w835:cluster{"Name":string, "Value":dbl}[])  [unwired: 1 in, 8 out]
        n382 = call "Actuator Data Set.vi"("Selected LBCB"=w818, "Measurement Actions"=Actuator_Measurment_Actions."Get") -> ("Actuator Data Out"=w832:T56)  [unwired: 3 in, 6 out]
        n383 = Unbundle By Name(w832) -> ("Commands"=w825:dbl[])
        n384 = call "Generate Data Tables.vi"("LBCB Number"=w818, "Cartesian Type"=w836) -> ("Actuator Table"=w838:dbl[][], "Cartesian Table"=w837:dbl[][])  [unwired: 3 out]
        n385 = local write "External Sensors"(w835) -> ()
        n386 = local write "Cartesian Digital Display Table"(w837) -> ()
        n387 = local write "Actuator Digital Display"(w838) -> ()
        n388 = Index Array(array=w825, index #1=0, index #2=1, index #3=2, index #4=3, index #5=4, index #6=5) -> (element #1=w824:dbl, element #2=w823:dbl, element #3=w822:dbl, element #4=w821:dbl, element #5=w820:dbl, element #6=w819:dbl)
        n389 = local write "Actuator X1"(w824) -> ()
        n390 = local write "Actuator X2"(w823) -> ()
        n391 = local write "Actuator Y1"(w822) -> ()
        n392 = local write "Actuator Z1"(w821) -> ()
        n393 = local write "Actuator Z2"(w820) -> ()
        n394 = local write "Actuator Z3"(w819) -> ()
      }
      frame #2 {
        # "There may be a problem with Hold Measurements calling\nCartesian Data Set too often"
        n395 = Wait on Notification(notifier=w847, timeout in ms (-1)=w840, error in (no error)=w846) -> (notifier out=w845:refnum<notifier>, notification=w842:T25, timed out?=w843:bool, error out=w844:errorcluster)  [unwired: 1 out]
        n396 = case shown="False" w843 {
          tunnel: w842 -> [w864 _]
          tunnel: w841 -> [w849 _]
          tunnel: w839 -> [w857 _]
          frame #0 {
            n397 = Unbundle By Name(w864) -> ("LBCB Target"=w863:T17[], "LBCB Convergence"=w862:T15[], "MixedModeStates"=→"MixedModeStates":T19)
            n398 = call "Get Hold Measurements.vi"("Use Offsets"=w857, "LBCB Number"=w849) -> ("Measurements"=w856:T16)  [unwired: 9 in]
            n399 = Index Array(array=w863, index=w849) -> (element=w861:T17)
            n400 = Index Array(array=w862, index=w849) -> (element=w860:T15)
            n401 = call "MM Multi DOF Status DAO.vi"("Actions"=DAO_Actions."Get") -> ("Mixed Mode Multidof Status Out"=w853:T57)  [unwired: 9 in, 1 out]
            n402 = call "Calculated Stiffness Jacobian.vi"("LBCB Number"=w849, "Actions"=Persistant_DAO_Actions."Get") -> ("Stiffness Jacobian Out"=w859:T18)  [unwired: 2 in, 7 out]
            n403 = Unbundle By Name(w853) -> ("Mixed Mode Multidof State"=w852:T20, "Multi DOF Ramp Count"=w851:i32, "Stiffness Tested"=w850:T1[][])
            n404 = local write "Measurements"(w856) -> ()
            n405 = local write "Convergence"(w860) -> ()
            n406 = local write "Target"(w861) -> ()
            n407 = local write "Stiffness Jacobian"(w859) -> ()
            n408 = Index Array(array=w850, index (row)=w849) -> (element=w848:T1[])  [unwired: 1 in]
            n409 = local write "Mixed Mode Multidof State"(w852) -> ()
            n410 = local write "MM Multi Ramp Count"(w851) -> ()
            n411 = local write "Stiffness Tested"(w848) -> ()
          }
          frame #1 {
          }
        }
      }
      frame #3 {
        n412 = Wait Until Next ms Multiple(millisecond multiple=w867) -> ()  [unwired: 1 out]
        n413 = call "Autobalance Data DAO.vi"("DAO Actions"=DAO_Actions."Get") -> ("L2 Autobalance Out"=w870:T58[], "L1 Autobalance Out"=w871:T58[])  [unwired: 3 in, 6 out]
        n414 = Select(t=w870, s=w872, f=w871) -> (s? t:f=w869:T58[])
        n415 = call "AB Status 2 AB Display Status.vi"("Autobalance Status In"=w869) -> ("Autobalance Statuses Out"=w868:T23[])  [unwired: 10 in]
        n416 = local write "Autobalance Statuses"(w868) -> ()
      }
    }
  }
  n417 = Compound Arithmetic op=AND(w32, w24, w23, w8) -> (w22:bool)
  "all stopped" <- w22
  n418 = Not(x=w22) -> (.not. x?=w21:bool)
  n419 = flat-sequence {
    tunnel: w21 -> [w876]
    frame #0 {
      n420 = local write "stop"(w876) -> ()
      n421 = control-ref of="This VI"() -> (w874:refnum<vi>)
      n422 = property on="Fake" class="Bool (strict)"("Visible"=TRUE) -> ()  [unwired: 2 in, 2 out]
      n423 = invoke class="VI" method="FP.Close"(reference=w874) -> ()  [unwired: 2 in, 3 out]
    }
  }
